vi "Module - Developer.vi"(11 "Stop":bool) -> (0 "Error Out":errorcluster)   [LabVIEW 2020]
uses:
  Control/Header - Select List Module.ctl
  Control/State - Module Developer.ctl
  <vilib>/Utility/miscctls.llb/LVPointTypeDef.ctl
  <vilib>/Utility/miscctls.llb/LVRowAndColumnUnsignedTypeDef.ctl
  <vilib>/Utility/miscctls.llb/LVPositionTypeDef.ctl
  <vilib>/Utility/miscctls.llb/LVRowAndColumnTypeDef.ctl
  Control/State - eFGV.ctl
  Control/Page List Configuration.ctl
  <vilib>/Utility/sysdir.llb/System Directory Type.ctl
  4b85dc79-c13a-48f8-9fb5-d693e32ae90e.vi
  de5a3265-ad59-4465-a9dd-367ad4980a1d.vi
  9e867a0b-6b5b-460c-ac8a-66f89ab5f6ca.vi
  ea73c07c-52c5-4c90-b3f8-ef615bf6d849.vi
  6d7569e3-b217-40ce-8343-143ededf8619.vi
  <vilib>/Utility/file.llb/Read Delimited Spreadsheet (string).vi
panel:
  in  "Page":enum32{"Page 1", "Page 2", "Page 3", "Page 4"}(radio)
  in  "Refresh":bool
  out "Max":i32
  in  "RT: Select All List":bool caption="Select All"
  in  "RT: Select All Module":bool caption="Select All"
  in  "Tab Control":enum32{"Page 1", "Page 2", "Page 3", "Page 4"}(tab)
  in  "HMI: Project Name":string caption="Project Name:"
  in  "HMI State":T1(ring)=enum."Maximized"
  in  "HMI: Check License":bool caption="Check License"
  in  "HMI: EXE Name":string caption="EXE Name:"
  in  "Page List":i32(listbox)
  in  "HMI: Version":enum16{"Demo", "User"}(ring) caption="Version"
  in  "HMI: Min Page":i32=2 caption="Minimum Page" min=2 max=8
  in  "HMI: Max Page":enum16{"4", "5", "6", "7", "8", "9"}(ring) caption="Maximum Page"
  out "No":i32[](array[numeric])=[1, 2, 3, 4, 5, 6, 7, 8, 9, 10, 11, 12, 13, 14, 15, 16, 17, 18, 19, 20, 21, 22, 23, 24, 25]
  in  "Res: Width":i16=1356
  in  "Res: Height":i16=655
  in  "Font Size":u32=44
  in  "License Level":T2(ring)=enum."Level 2"
  in  "License Type":T3(ring)=enum."Perpetual"
  in  "HMI: Default":bool
  in  "HMI: Select List":T4=enum."2 Default Run Module" caption="Select List"
  in  "Tip Strip":string caption="Set Button Tip Strip"
  in  "HMI: List":cluster{"Module Name":string, "Selected":bool}[](array[cluster])
  in  "Text":string caption="Set Button Text"
  in  "HMI: Update Text":bool
  in  "Table: Button Text":i32(listbox)
  in  "HMI: Down":bool
  in  "HMI: Up":bool
  in  "HMI: Sort":bool
  in  "HMI: Add":bool
  in  "HMI: Remove":bool
  in  "HMI: All Module":cluster{"Module Name":string, "Selected":bool}[](array[cluster]) caption="All Module"
  in  "HMI: Select All Module":bool caption="Select All"
  in  "RT: All Module":cluster{"Module Name":string, "Selected":bool}[](array[cluster])
  in  "RT: List":cluster{"Module Name":string, "Selected":bool}[](array[cluster])
  in  "RT: Add":bool
  in  "RT: Remove":bool
  in  "RT: Up":bool
  in  "RT: Down":bool
  in  "Load Error":bool
  in  "Error Table":i32(listbox) caption="List of Error"
  # "Page List"
  # "General Setting"
  # "Configure List of HMI Module"
  # "Configure Button Text"
  # "Maximum 15 page configurable"
  # "Configure List of RT Engine Module"
  # "Error Management"
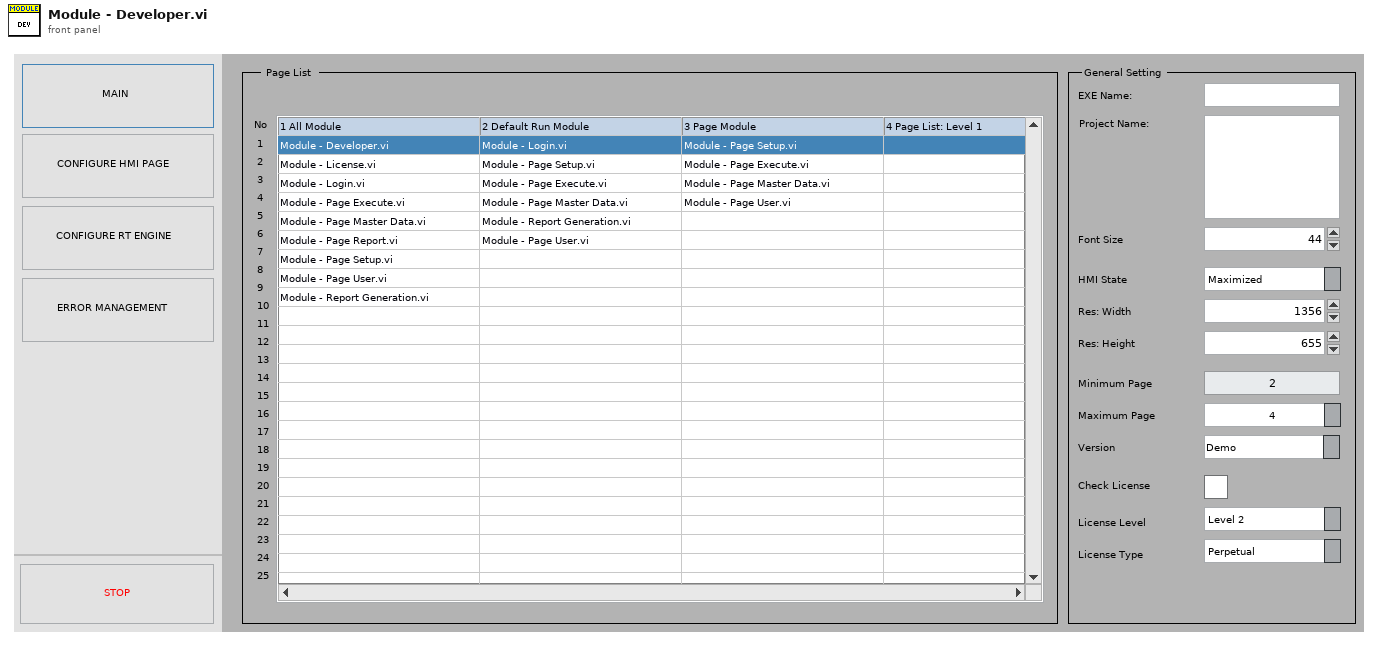
[diagram p1: front panel]
types:
  T1 = enum32{"Invalid", "Standard", "Closed", "Hidden", "Minimized", "Maximized"}
  T2 = enum32{"Level 1", "Level 2", "Level 3", "Level 4", "Level 5"}
  T3 = enum32{"Free", "Trial", "Subscription", "Perpetual"}
  T4 = typedef "Header - Select List Module.ctl" = enum16{"1 All Module", "2 Default Run Module", "3 Page Module", "4 Page List: Level 1", "5 Page List: Level 2", "6 Page List: Level 3", "7 All RT Module", "8 Default RT Run Module", "9 Acquire Enable Page", "10 Log Enable Page", "11 Run Page", "12 Kill Page", "13 Button Text", "14 Button Tip Strip"}
  T5 = cluster{"HMI?":bool, "HMI":cluster{"Button Ref":refnum<vi>[], "All Module":string[], "Button Disabled":enum8{"Enabled", "Disabled", "Disabled and Grayed Out"}[], "List From":enum16{"All HMI", "List HMI"}, "List Select":bool[]}, "RT":cluster{"Button Ref":refnum<vi>[], "All Module":string[], "Button Disabled":enum8{"Enabled", "Disabled", "Disabled and Grayed Out"}[], "List From":enum16{"All RT", "List RT"}, "List Select":bool[]}, "Event Ref":refnum<event-registration>}
  T6 = typedef "State - Module Developer.ctl" = enum16{"Init", "Register Event", "Get All Module", "Populate Page List", "Populate RT Module", "Idle", "HMI: List Disable", "HMI: Button Disable", "HMI: Update List", "HMI: Update Text Button", "HMI: Add to List", "HMI: Remove from List", "HMI: Sort List", "HMI: Up List", "HMI: Down List", "HMI: Set Default List", "RT: Add to List", "RT: Remove from List", "RT: Up List", "RT: Down List", "RT: List Disable", "RT: Button Disable", "Update Page List", "Save Page List", "Load Error", "Close"}
  T7 = typedef "LVPointTypeDef.ctl" = cluster{"Horizontal":i16, "Vertical":i16}
  T8 = typedef "LVPositionTypeDef.ctl" = cluster{"Left":i32, "Top":i32}
  T9 = typedef "LVRowAndColumnUnsignedTypeDef.ctl" = cluster{"Row":u32, "Column":u32}
  T10 = typedef "LVRowAndColumnTypeDef.ctl" = cluster{"Row":i32, "Column":i32}
  T11 = typedef "State - eFGV.ctl" = enum16{"Init", "Read", "Write", "Exit"}
  T12 = enum16{"Always On", "Always Off", "Off While Running"}
  T13 = enum8{"Enabled", "Disabled", "Disabled and Grayed Out"}
  T14 = typedef "Page List Configuration.ctl" = cluster{"HMI Configuration":cluster{"EXE Name":string, "Project Name":string, "Max Page No":i32, "HMI State":enum32{"Invalid", "Standard", "Closed", "Hidden", "Minimized", "Maximized"}, "Version":enum16{"Demo", "User"}, "Check License":bool, "Font Size":u32, "Res: Height":i16, "Res: Width":i16, "License Level":enum16{"Level 1", "Level 2", "Level 3", "Level 4", "Level 5"}, "License Type":enum16{"Free", "Trial", "Subscription", "Perpetual"}}, "All HMI Module":string[], "Default HMI Module":string[], "Page Module":string[], "Page List: Level 1":string[], "Page List: Level 2":string[], "Page List: Level 3":string[], "All RT Module":string[], "Default RT Module":string[], "Acquire Enable Page":string[], "Log Enable Page":string[], "Run Page":string[], "Kill Page":string[], "Button":cluster{"Text":string[], "Tip Strip":string[]}}
  T15 = enum32{"invalid app kind", "Development System", "Run Time System", "Student Edition", "Embedded LabVIEW", "Evaluation", "Custom"}
  T16 = enum16{"Free", "Trial", "Subscription", "Perpetual"}
  T17 = enum16{"Level 1", "Level 2", "Level 3", "Level 4", "Level 5"}
  T18 = enum8{"Enabled", "Disabled", "Disabled and Grayed Out"}[]
  T19 = typedef "System Directory Type.ctl" = i32
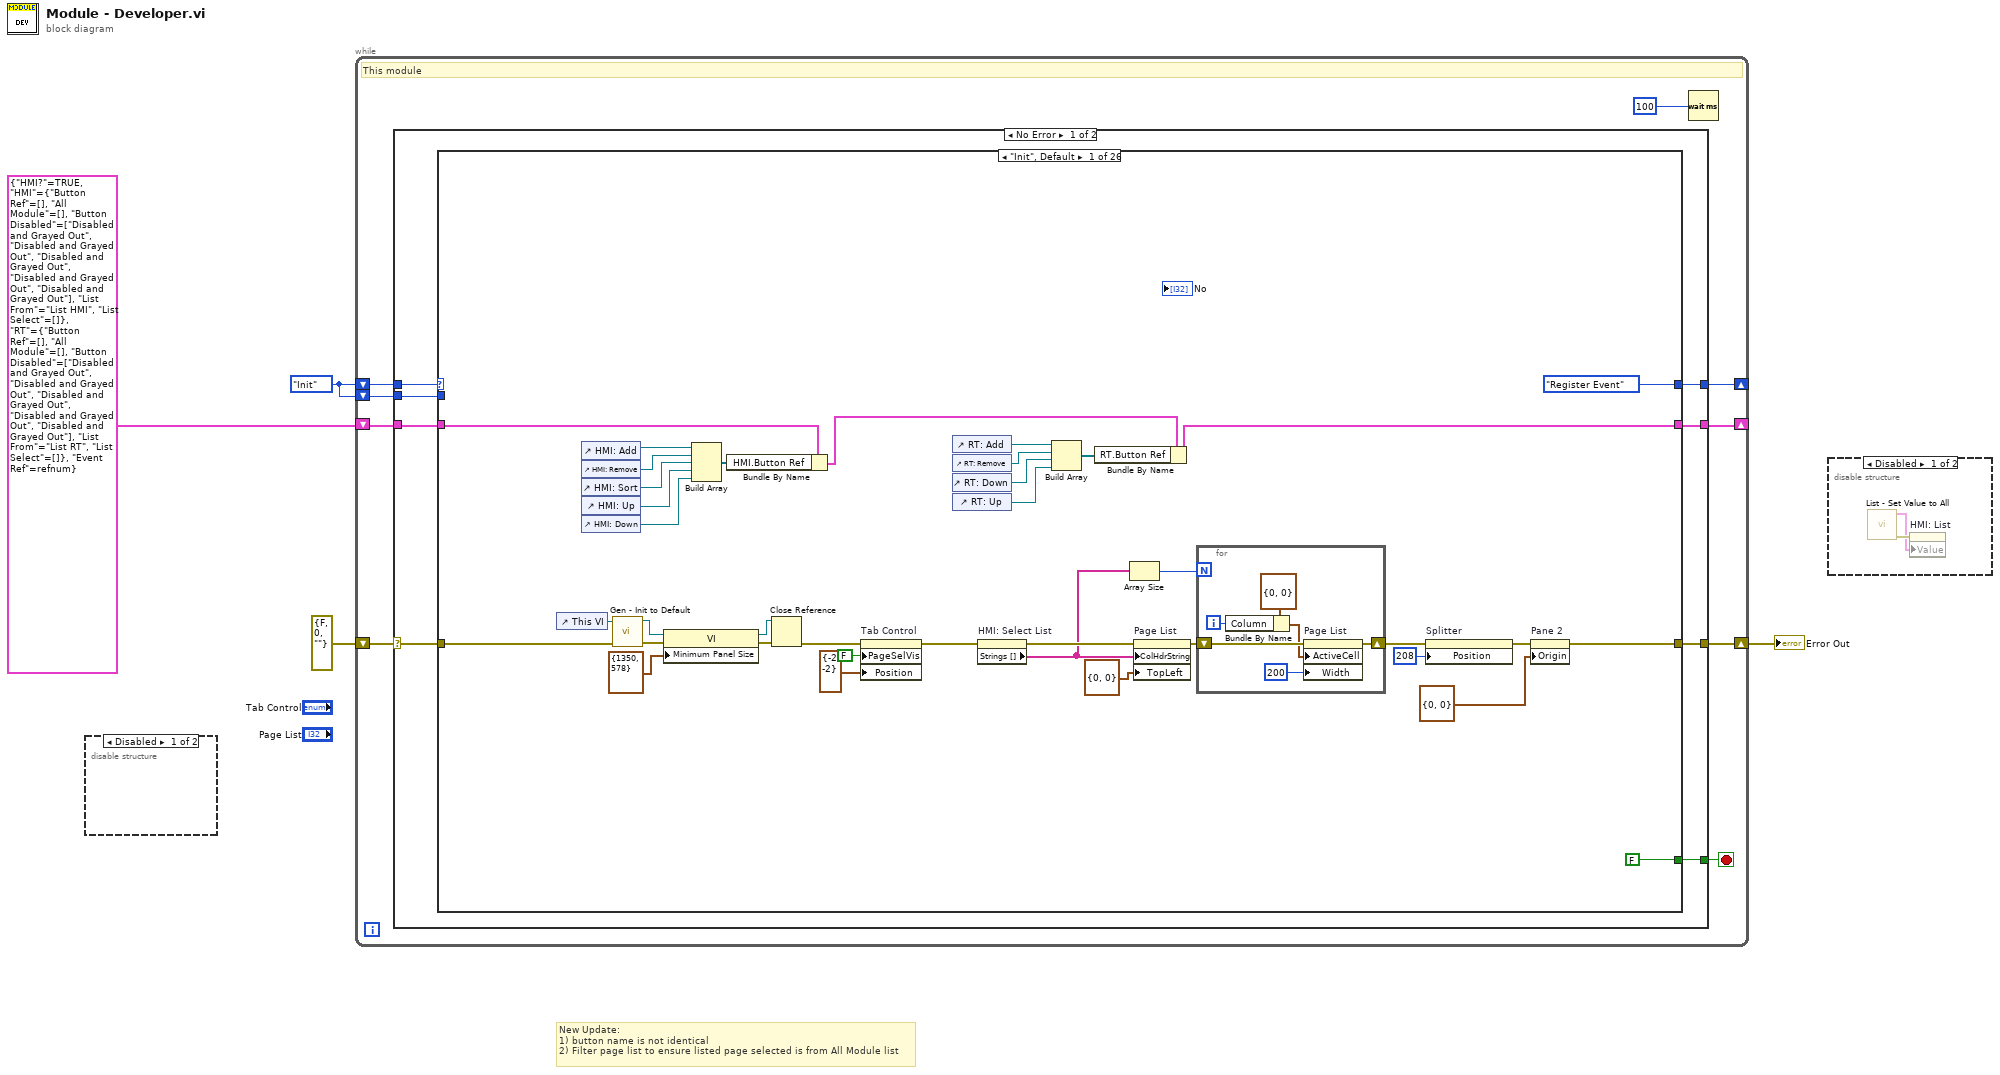
[diagram p0: block diagram]
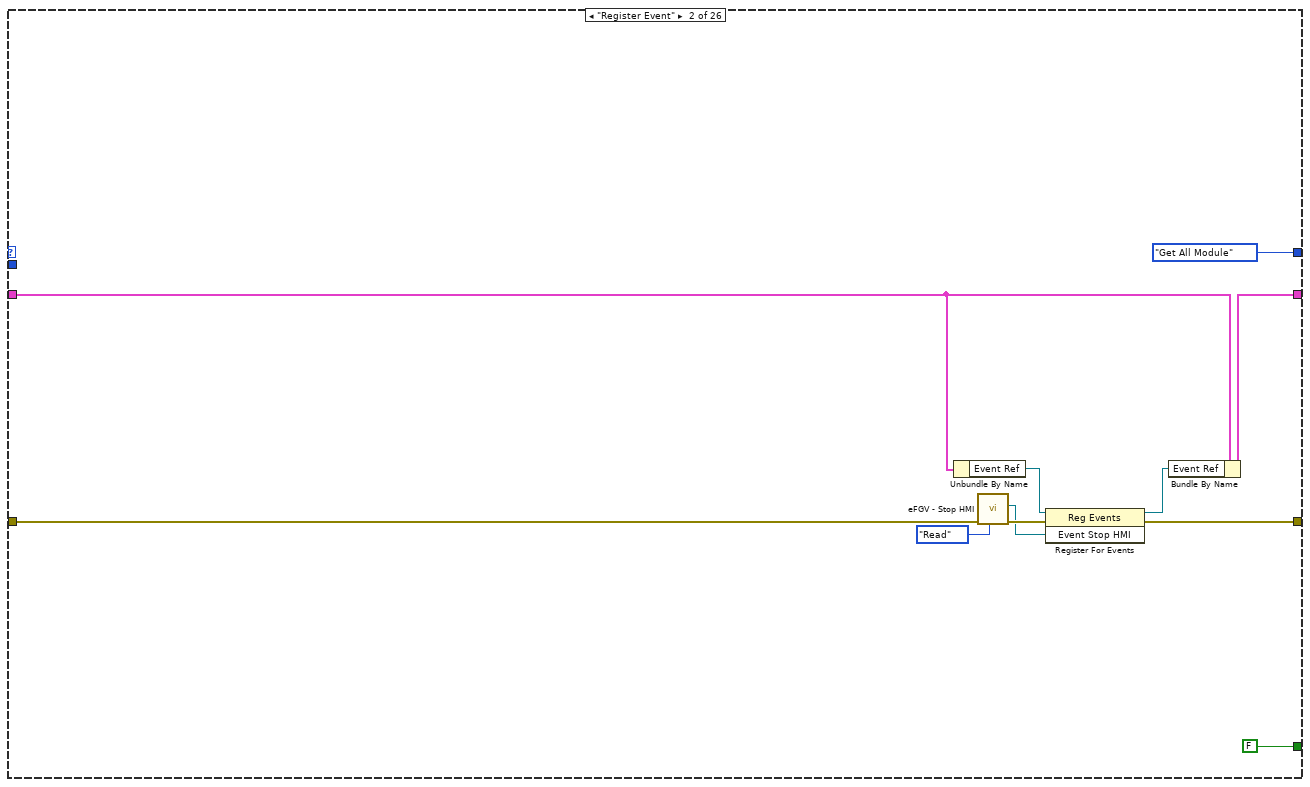
[diagram p4: hidden frame]
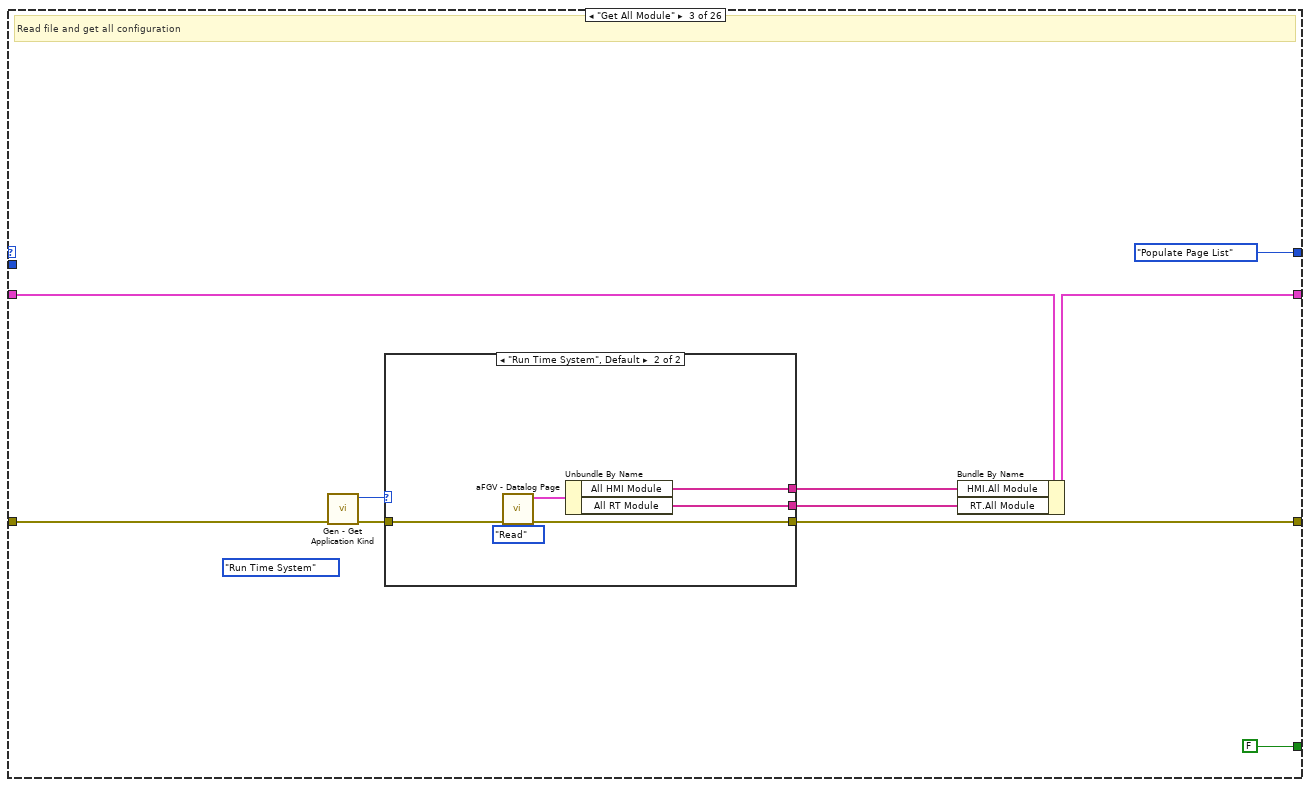
[diagram p5: hidden frame]
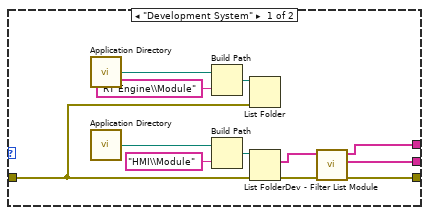
[diagram p6: hidden frame]
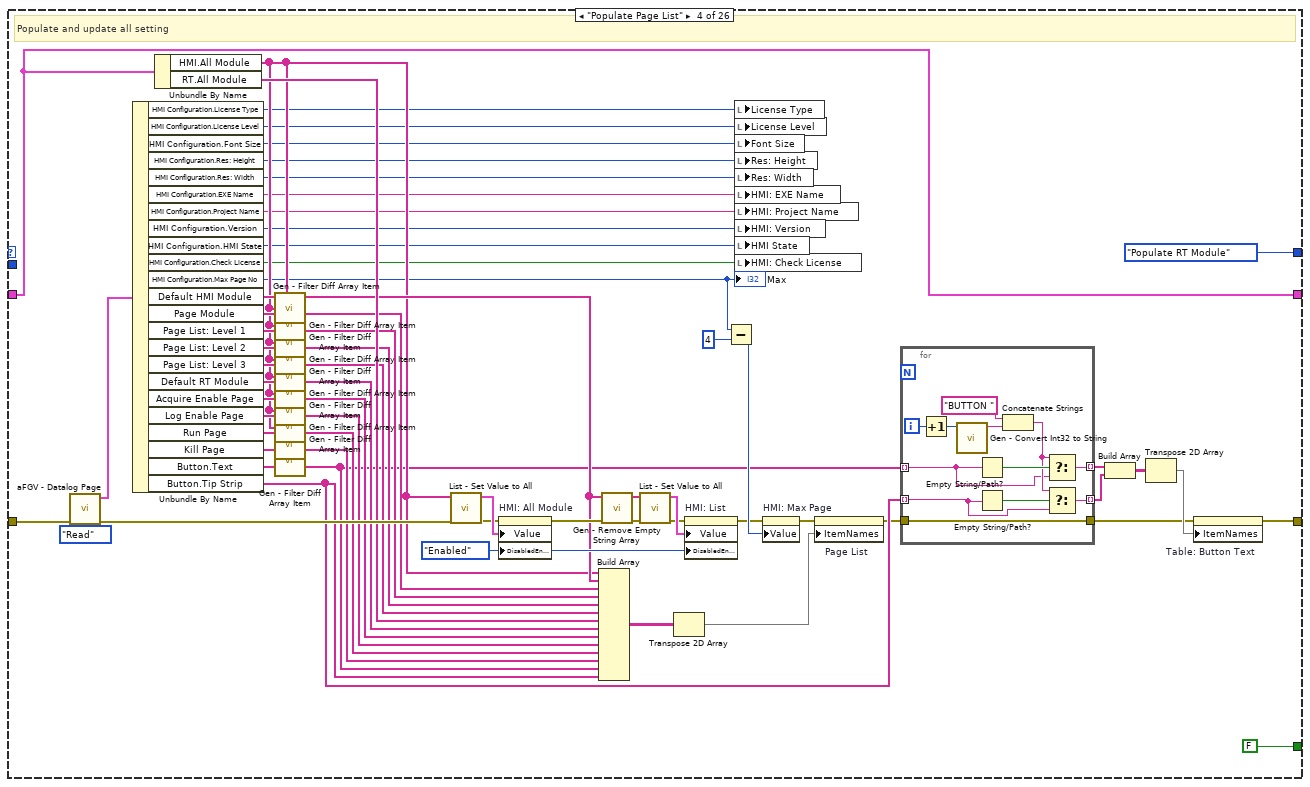
[diagram p7: hidden frame]
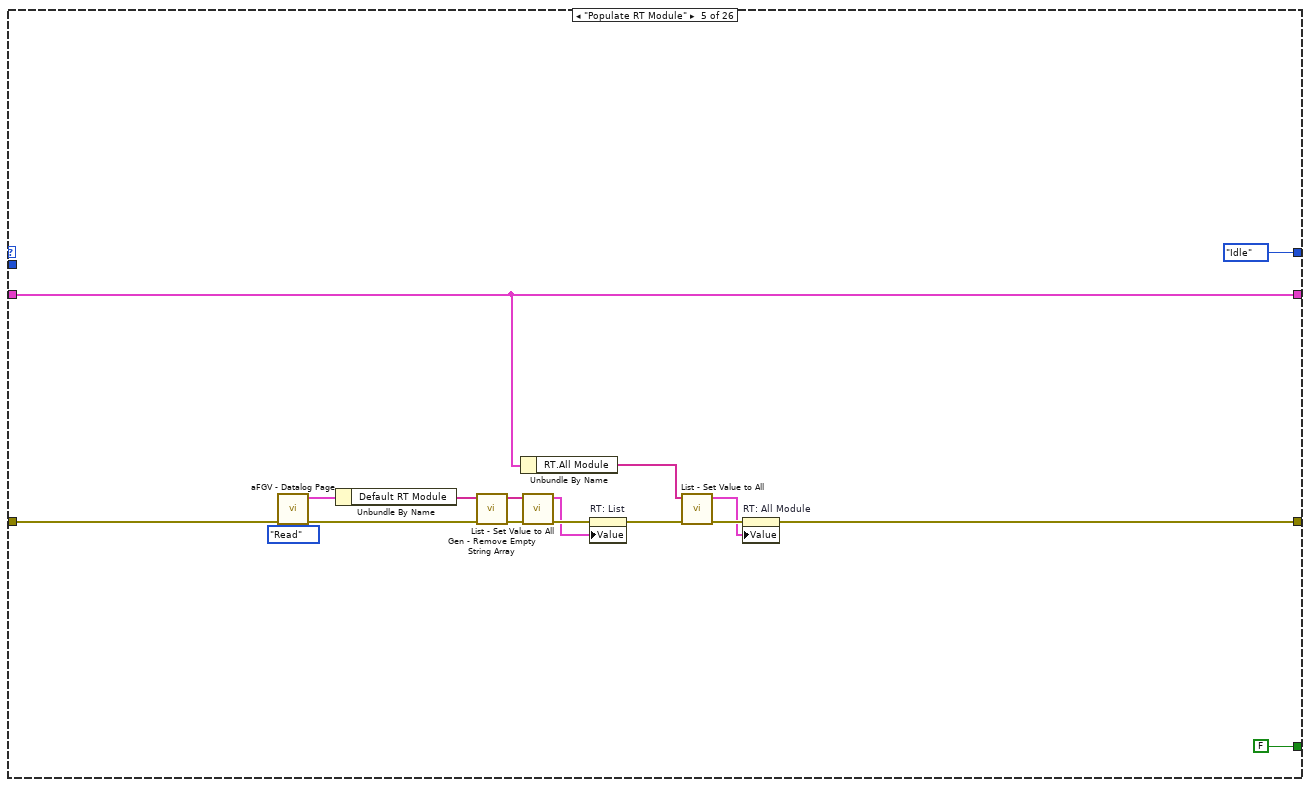
[diagram p8: hidden frame]
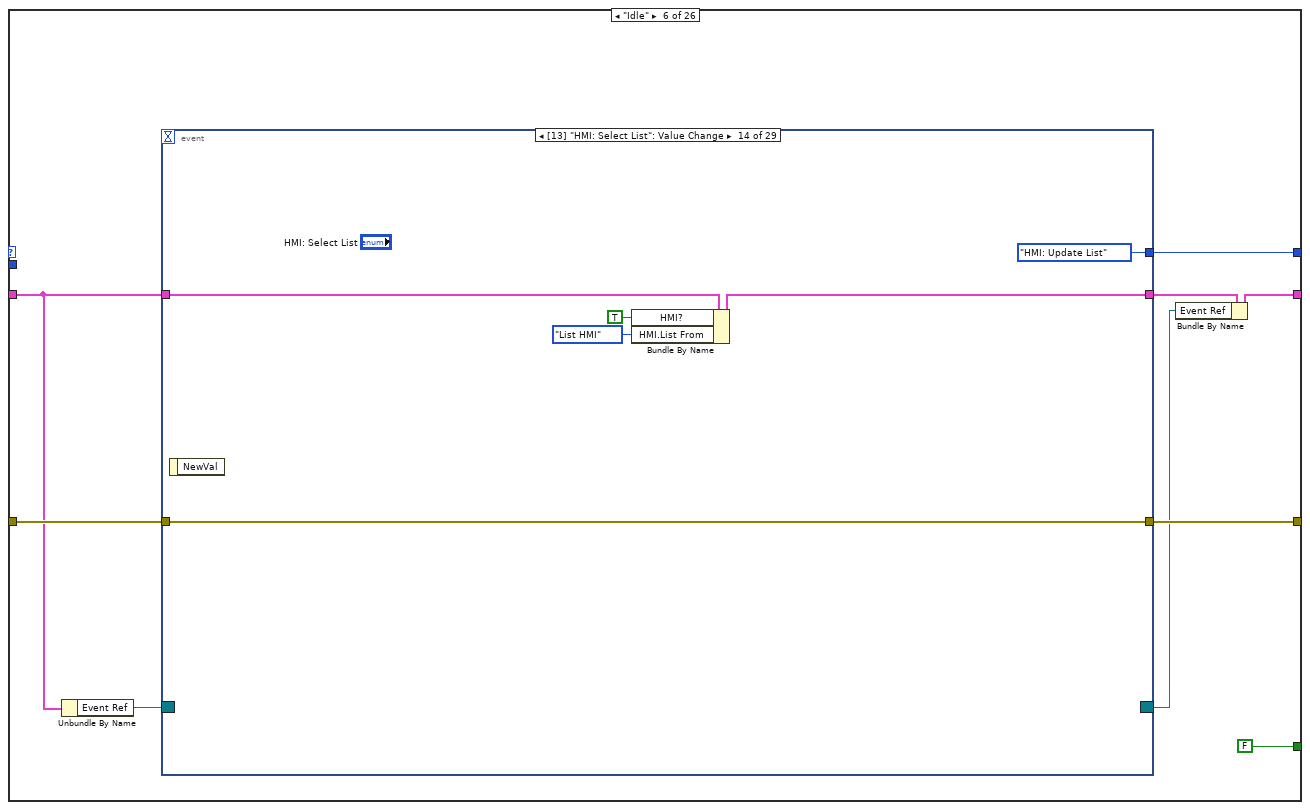
[diagram p9: hidden frame]
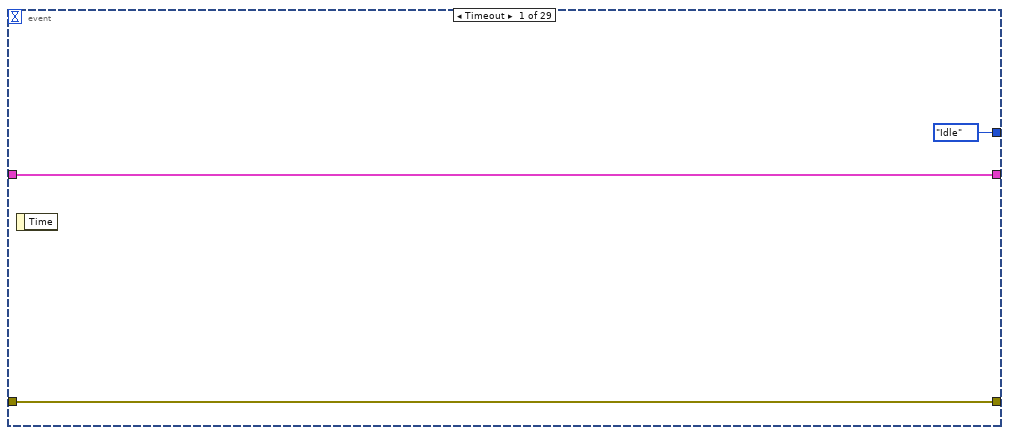
[diagram p10: hidden frame]
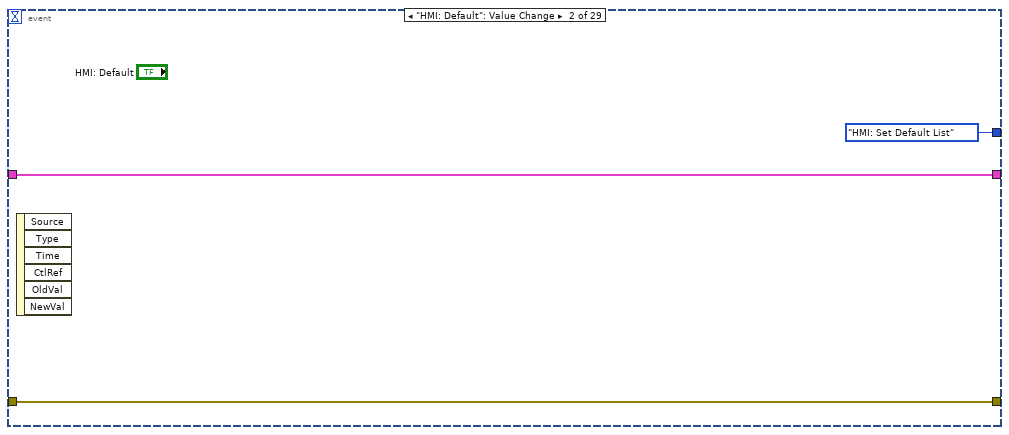
[diagram p11: hidden frame]
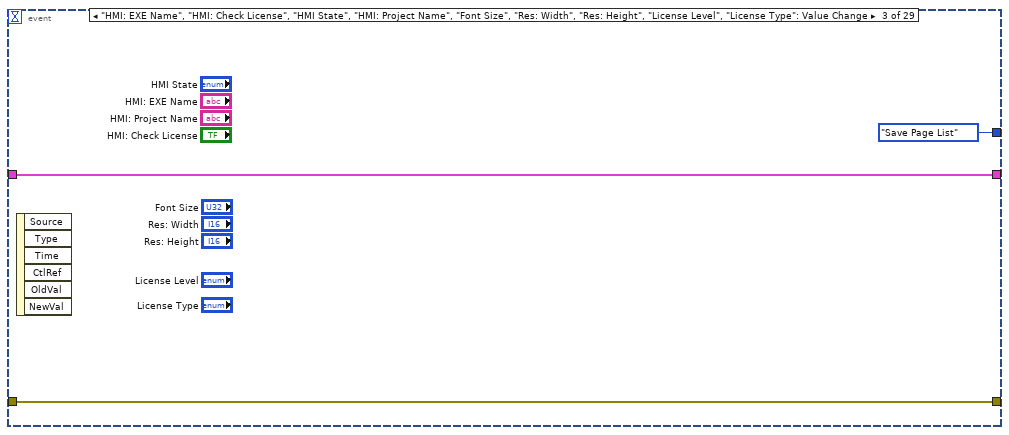
[diagram p12: hidden frame]
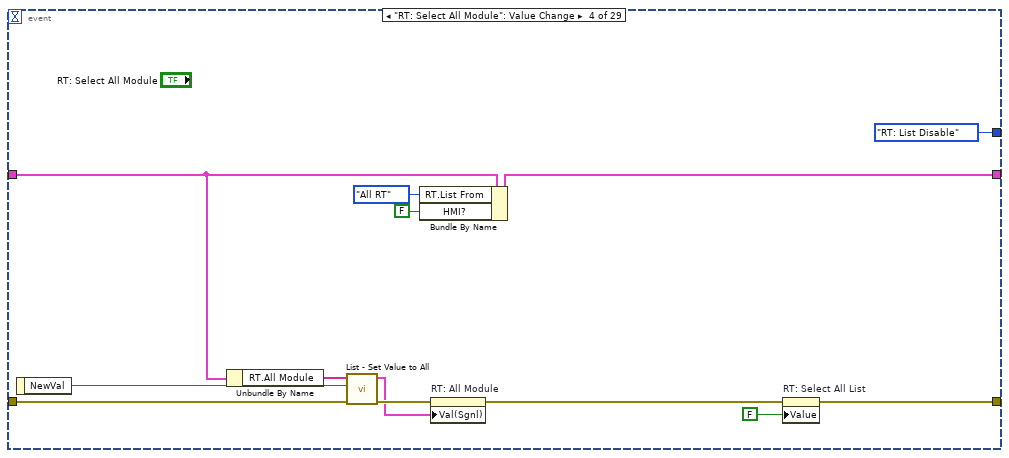
[diagram p13: hidden frame]
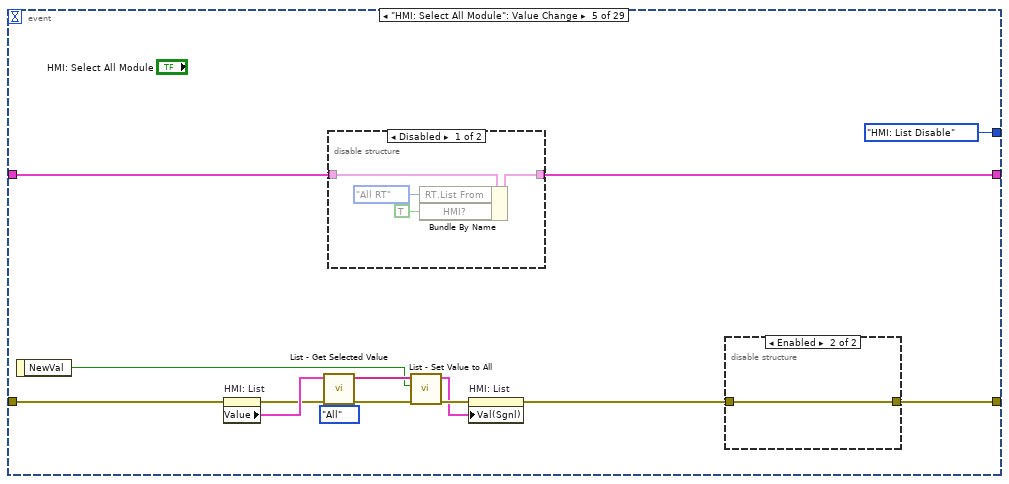
[diagram p14: hidden frame]
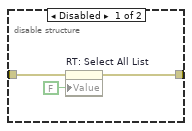
[diagram p15: hidden frame]
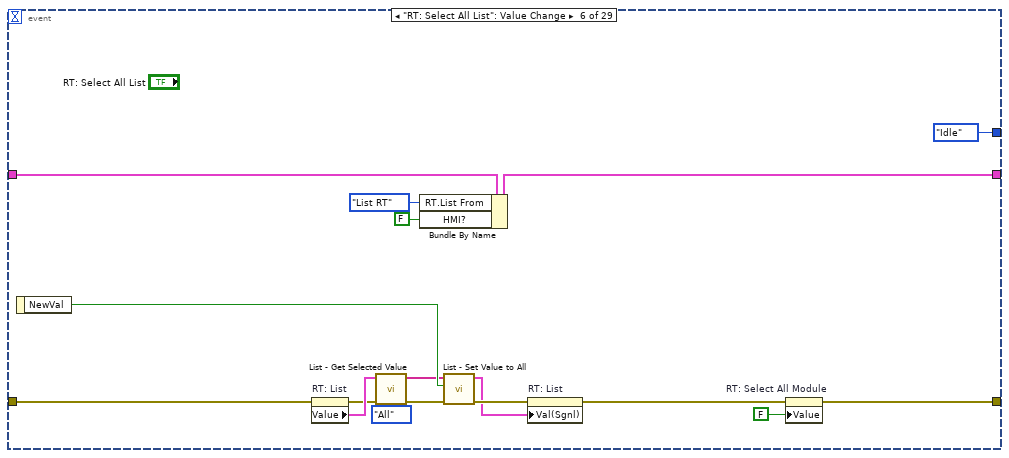
[diagram p17: hidden frame]
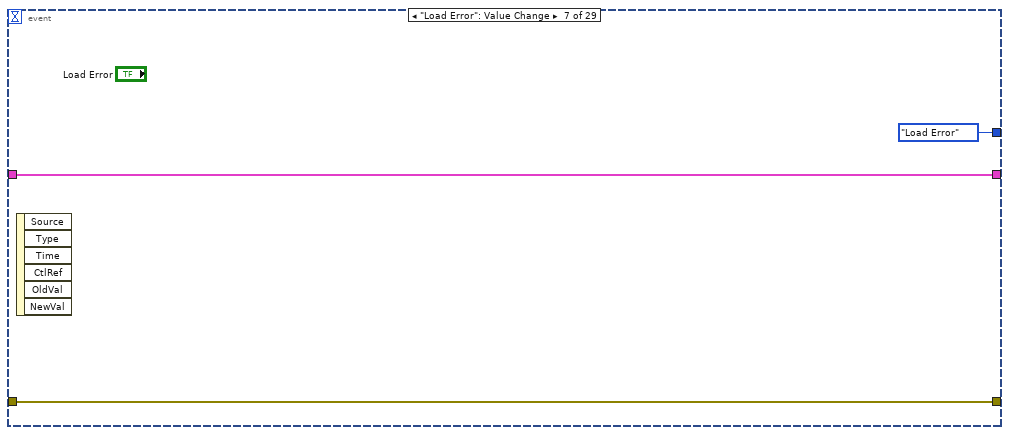
[diagram p18: hidden frame]
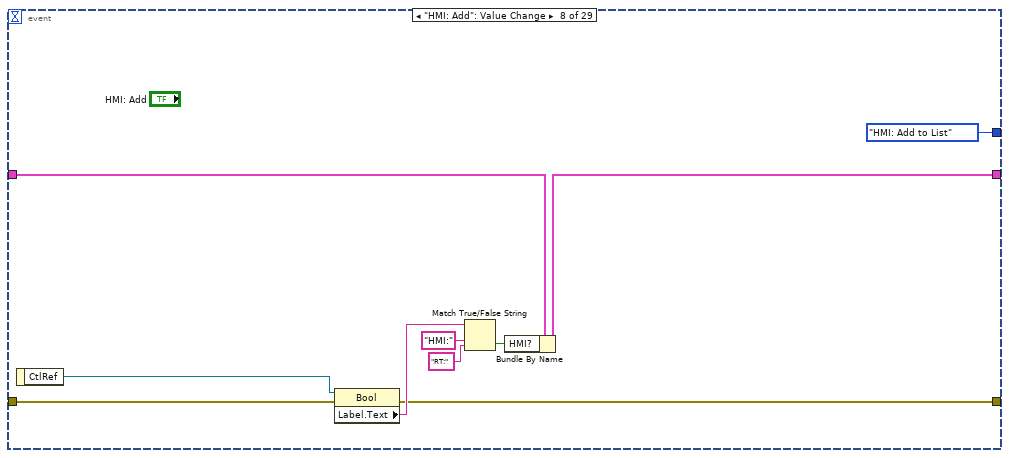
[diagram p19: hidden frame]
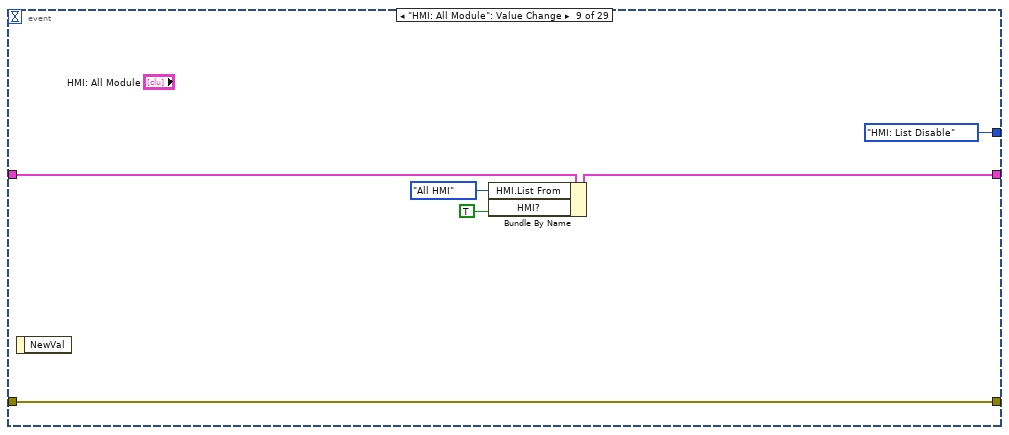
[diagram p20: hidden frame]
diagram:
  w1 = State_-_Module_Developer."Init"
  # "New Update:\n1) button name is not identical\n2) Filter page list to ensure listed page selected is from All Module list"
  n1 = disable-structure shown="Disabled" {
    frame Disabled {
    }
    frame Enabled {
    }
  }
  n2 = while {
    shift-right: [w9] -> _
    shift-left: w1 -> [w11]
    shift-right: [w12] -> w3
    shift-left: errorcluster {"status"=FALSE, "code"=0, "source"=""} ("Error In") -> [w13]
    shift-right: [w7] -> _
    shift-left: T5 {"HMI?"=TRUE, "HMI"={"Button Ref"=[], "All Module"=[], "Button Disabled"=[enum."Disabled and Grayed Out", enum."Disabled and Grayed Out", enum."Disabled and Grayed Out", enum."Disabled and Grayed Out", enum."Disabled and Grayed Out"], "List From"=enum."List HMI", "List Select"=[]}, "RT"={"Button Ref"=[], "All Module"=[], "Button Disabled"=[enum."Disabled and Grayed Out", enum."Disabled and Grayed Out", enum."Disabled and Grayed Out", enum."Disabled and Grayed Out", enum."Disabled and Grayed Out"], "List From"=enum."List RT", "List Select"=[]}, "Event Ref"=refnum} -> [w8]
    shift-left: w1 -> [w5]
    stop <- w10 stop-if-true
    # "This module"
    n3 = case shown="No Error" w13 {
      selector: w13 -> [w20 w1068]
      tunnel: w11 -> [w19 w1070]
      tunnel: [w21 w1067] -> w12
      tunnel: [w18 FALSE] -> w10
      tunnel: [w17 w1070] -> w9
      tunnel: w8 -> [w16 w1069]
      tunnel: [w15 w1069] -> w7
      tunnel: w5 -> [w14 _]
      frame No Error {
        n4 = case shown="\"Init\", Default" w19 {
          tunnel: [w32 w75 w82 w149 w178 w202 w440 w496 w530 w565 w639 w649 w674 w685 w710 w725 w766 w775 w784 w809 w822 w900 w923 w1015 w1019 w1056] -> w21
          tunnel: w20 -> [w58 w73 w79 w156 w190 w201 w439 w489 w529 w580 w633 w657 w675 w695 w714 w724 w758 w776 w794 w813 w834 w878 w908 w957 w1020 w1061]
          tunnel: [FALSE FALSE FALSE FALSE FALSE FALSE FALSE FALSE FALSE FALSE FALSE FALSE FALSE FALSE FALSE FALSE FALSE FALSE FALSE FALSE FALSE FALSE FALSE FALSE FALSE TRUE] -> w18
          tunnel: [State_-_Module_Developer."Register Event" State_-_Module_Developer."Get All Module" State_-_Module_Developer."Populate Page List" State_-_Module_Developer."Populate RT Module" State_-_Module_Developer."Idle" w199 State_-_Module_Developer."HMI: Button Disable" State_-_Module_Developer."Idle" State_-_Module_Developer."HMI: List Disable" State_-_Module_Developer."Save Page List" State_-_Module_Developer."Update Page List" State_-_Module_Developer."Update Page List" State_-_Module_Developer."Save Page List" State_-_Module_Developer."Update Page List" State_-_Module_Developer."Update Page List" State_-_Module_Developer."Update Page List" State_-_Module_Developer."Update Page List" State_-_Module_Developer."Update Page List" State_-_Module_Developer."Update Page List" State_-_Module_Developer."Update Page List" State_-_Module_Developer."RT: Button Disable" State_-_Module_Developer."Idle" State_-_Module_Developer."Save Page List" w953 State_-_Module_Developer."Idle" State_-_Module_Developer."Close"] -> w17
          tunnel: w16 -> [w57 w68 w85 w148 w189 w197 w454 w495 w539 w588 w640 w664 w681 w700 w722 w743 w769 w783 w799 w821 w847 w899 w928 w1017 w1033 w1055]
          tunnel: [w27 w66 w81 w148 w189 w195 w436 w495 w539 w588 w640 w664 w681 w700 w722 w743 w769 w783 w799 w821 w831 w899 w928 w1017 w1033 w1055] -> w15
          tunnel: w14 -> [_ _ _ _ _ _ _ _ _ _ _ _ _ _ _ _ _ _ _ _ _ _ _ _ _ _]
          frame "Init", Default {
            n5 = control-ref of="This VI"() -> (w51:refnum<vi>)
            n6 = control-ref of="HMI: Add"() -> (w50:refnum<vi>)
            n7 = control-ref of="HMI: Remove"() -> (w49:refnum<vi>)
            n8 = control-ref of="HMI: Sort"() -> (w48:refnum<vi>)
            n9 = control-ref of="HMI: Up"() -> (w47:refnum<vi>)
            n10 = control-ref of="HMI: Down"() -> (w46:refnum<vi>)
            n11 = call "Gen - Init to Default.vi"("Error in"=w58, "This VI"=w51) -> ("Error out"=w33:errorcluster, "This VI Copy"=w34:refnum<vi>)  [unwired: 8 in]
            n12 = property class="VI"(reference=w34, error in=w33, "Minimum Panel Size"=T7 {"Horizontal"=1350, "Vertical"=578} ("Front Panel Window:Minimum Size")) -> (reference out=w36:refnum<vi>, error out=w37:errorcluster)
            n13 = Build Array(w50, w49, w48, w47, w46) -> (w44:refnum<vi>[])
            n14 = Bundle By Name(cluster=w57, "HMI.Button Ref"=w44) -> (w45:T5)
            n15 = Close Reference(reference=w36, error in (no error)=w37) -> (error out=w23:errorcluster)
            n16 = property on="Tab Control" class="TabCtl (strict)"(error in=w23, "PageSelVis"=FALSE ("Page Selector Visible"), "Position"=T8 {"Left"=-2, "Top"=-2}) -> (error out=w22:errorcluster)  [unwired: 1 in, 1 out]
            n17 = control-ref of="RT: Add"() -> (w31:refnum<vi>)
            n18 = control-ref of="RT: Remove"() -> (w30:refnum<vi>)
            n19 = control-ref of="RT: Down"() -> (w29:refnum<vi>)
            n20 = control-ref of="RT: Up"() -> (w28:refnum<vi>)
            n21 = property on="HMI: Select List" class="Enum (strict)"(error in=w22) -> (error out=w25:errorcluster, "Strings []"=w24:string[])  [unwired: 1 in, 1 out]
            n22 = Build Array(w31, w30, w29, w28) -> (w26:refnum<vi>[])
            n23 = Bundle By Name(cluster=w45, "RT.Button Ref"=w26) -> (w27:T5)
            n24 = Array Size(array=w24) -> (size(s)=w42:i32)
            n25 = property on="Page List" class="MCListbox (strict)"(error in=w25, "ColHdrString"=w24, "TopLeft"=T9 {"Row"=0, "Column"=0} ("Top Left Visible Cell")) -> (error out=w43:errorcluster)  [unwired: 1 in, 1 out]
            n26 = for {
              N: w42 -> [_]
              shift-right: [w63] -> w41
              shift-left: w43 -> [w64]
              i -> [w60]
              n27 = Bundle By Name(cluster=T10 {"Row"=0, "Column"=0} ("Active Cell:Active Cell"), "Column"=w60) -> (w61:T10)
              n28 = property on="Page List" class="MCListbox (strict)"(error in=w64, "ActiveCell"=w61, "Width"=u32 200 ("Active Cell:Cell Size:Width")) -> (error out=w63:errorcluster)  [unwired: 1 in, 1 out]
            }
            n29 = property on="Splitter" class="Splitter"(error in=w41, "Position"=208 ("Splitter Position")) -> (error out=w53:errorcluster)  [unwired: 1 in, 1 out]
            n30 = property on="Pane 2" class="Pane"(error in=w53, "Origin"=T7 {"Horizontal"=0, "Vertical"=0}) -> (error out=w32:errorcluster)  [unwired: 1 in, 1 out]
          }
          frame "Register Event" {
            n31 = Unbundle By Name(w68) -> ("Event Ref"=w67:refnum<event-registration>)
            n32 = call "eFGV - Stop HMI.vi"("Action"=State_-_eFGV."Read", "Error In"=w73) -> ("Error Out"=w74:errorcluster, "Event Stop HMI"=w71:refnum<user-event>)  [unwired: 7 in, 1 out]
            n33 = register-events(reference=w67, error in=w74, w71) -> (reference out=w65:refnum<event-registration>, error out=w75:errorcluster)
            n34 = Bundle By Name(cluster=w68, "Event Ref"=w65) -> (w66:T5)
          }
          frame "Get All Module" {
            (unwired) T15."Run Time System" ("Application:Kind")
            # "Read file and get all configuration"
            n35 = call "Gen - Get Application Kind.vi"("Error In"=w79) -> ("Error Out"=w77:errorcluster, "Application:Kind"=w78:T15)  [unwired: 9 in]
            n36 = case shown="\"Run Time System\", Default" w78 {
              tunnel: [w86 w102] -> w82
              tunnel: w77 -> [w92 w103]
              tunnel: [w87 w99] -> w80
              tunnel: [w88 w98] -> w76
              frame "Development System" {
                n37 = call <vilib>:"Application Directory.vi"() -> ("Application Directory"=w94:path)
                n38 = call <vilib>:"Application Directory.vi"() -> ("Application Directory"=w95:path)
                n39 = Build Path(base path=w94, name or relative path="RT Engine\\Module") -> (appended path=w93:path)
                n40 = Build Path(base path=w95, name or relative path="HMI\\Module") -> (appended path=w96:path)
                n41 = List Folder(path=w93, error in=w92) -> ()  [unwired: 2 in, 4 out]
                n42 = List Folder(path=w96, error in=w92) -> (filenames=w89:string[], error out=w90:errorcluster)  [unwired: 2 in, 2 out]
                n43 = call "Dev - Filter List Module.vi"("Error In"=w90, "Module In"=w89) -> ("Error Out"=w86:errorcluster, "RT Module"=w87:string[], "HMI Module"=w88:string[])  [unwired: 7 in]
              }
              frame "Run Time System", Default {
                n44 = call "aFGV - Datalog Page.vi"("Action"=enum16{"Read", "Write"}."Read", "Error In"=w103) -> ("Error Out"=w102:errorcluster, "Data Out"=w100:T14)  [unwired: 8 in]
                n45 = Unbundle By Name(w100) -> ("All HMI Module"=w98:string[], "All RT Module"=w99:string[])
              }
            }
            n46 = Bundle By Name(cluster=w85, "HMI.All Module"=w76, "RT.All Module"=w80) -> (w81:T5)
          }
          frame "Populate Page List" {
            w136 = T13."Enabled" ("Disabled")
            # "Populate and update all setting"
            n47 = call "aFGV - Datalog Page.vi"("Action"=enum16{"Read", "Write"}."Read", "Error In"=w156) -> ("Error Out"=w165:errorcluster, "Data Out"=w157:T14)  [unwired: 8 in]
            n48 = Unbundle By Name(w157) -> ("HMI Configuration.License Type"=w104:T16, "HMI Configuration.License Level"=w105:T17, "HMI Configuration.Font Size"=w108:u32, "HMI Configuration.Res: Height"=w107:i16, "HMI Configuration.Res: Width"=w106:i16, "HMI Configuration.EXE Name"=w114:string, "HMI Configuration.Project Name"=w113:string, "HMI Configuration.Version"=w112:enum16{"Demo", "User"}, "HMI Configuration.HMI State"=w111:T1, "HMI Configuration.Check License"=w109:bool, "HMI Configuration.Max Page No"=w110:i32, "Default HMI Module"=w134:string[], "Page Module"=w164:string[], "Page List: Level 1"=w163:string[], "Page List: Level 2"=w162:string[], "Page List: Level 3"=w161:string[], "Default RT Module"=w146:string[], "Acquire Enable Page"=w147:string[], "Log Enable Page"=w154:string[], "Run Page"=w153:string[], "Kill Page"=w152:string[], "Button.Text"=w122:string[], "Button.Tip Strip"=w121:string[])
            "Max" <- w110
            n49 = Unbundle By Name(w148) -> ("HMI.All Module"=w123:string[], "RT.All Module"=w135:string[])
            n50 = call "Gen - Filter Diff Array Item.vi"("All Element"=w123, "List in"=w134) -> ("List Out"=w133:string[])  [unwired: 9 in]
            n51 = call "Gen - Filter Diff Array Item.vi"("All Element"=w123, "List in"=w164) -> ("List Out"=w132:string[])  [unwired: 9 in]
            n52 = call "Gen - Filter Diff Array Item.vi"("All Element"=w123, "List in"=w163) -> ("List Out"=w131:string[])  [unwired: 9 in]
            n53 = call "Gen - Filter Diff Array Item.vi"("All Element"=w123, "List in"=w162) -> ("List Out"=w130:string[])  [unwired: 9 in]
            n54 = call "Gen - Filter Diff Array Item.vi"("All Element"=w123, "List in"=w161) -> ("List Out"=w129:string[])  [unwired: 9 in]
            n55 = call "Gen - Filter Diff Array Item.vi"("All Element"=w123, "List in"=w146) -> ("List Out"=w128:string[])  [unwired: 9 in]
            n56 = call "Gen - Filter Diff Array Item.vi"("All Element"=w123, "List in"=w147) -> ("List Out"=w127:string[])  [unwired: 9 in]
            n57 = call "Gen - Filter Diff Array Item.vi"("All Element"=w123, "List in"=w154) -> ("List Out"=w126:string[])  [unwired: 9 in]
            n58 = call "Gen - Filter Diff Array Item.vi"("All Element"=w123, "List in"=w153) -> ("List Out"=w125:string[])  [unwired: 9 in]
            n59 = call "Gen - Filter Diff Array Item.vi"("All Element"=w123, "List in"=w152) -> ("List Out"=w124:string[])  [unwired: 9 in]
            n60 = call "List - Set Value to All.vi"("Error In"=w165, "List In"=w123) -> ("Error Out"=w142:errorcluster, "List Out"=w143:cluster{"Name":string, "Selected":bool}[])  [unwired: 8 in]
            n61 = property on="HMI: All Module" class="Arr (strict)"(error in=w142, "Value"=w143, "DisabledEnum"=w136) -> (error out=w138:errorcluster)  [unwired: 1 in, 1 out]
            n62 = Build Array(w123, w133, w132, w131, w130, w129, w135, w128, w127, w126, w125, w124, w122, w121) -> (w155:string[][])
            n63 = call "Gen - Remove Empty String Array.vi"("Data Array"=w133) -> ("Data Out"=w141:string[])  [unwired: 10 in]
            n64 = call "List - Set Value to All.vi"("Error In"=w138, "List In"=w141) -> ("Error Out"=w139:errorcluster, "List Out"=w140:cluster{"Name":string, "Selected":bool}[])  [unwired: 8 in]
            n65 = Transpose 2D Array(2D array=w155) -> (transposed array=w151:string[][])
            n66 = property on="HMI: List" class="Arr (strict)"(error in=w139, "Value"=w140, "DisabledEnum"=w136) -> (error out=w137:errorcluster)  [unwired: 1 in, 1 out]
            n67 = Subtract(x=w110, y=4) -> (x-y=w145:i32)
            n68 = local write "License Type"(w104) -> ()
            n69 = local write "License Level"(w105) -> ()
            n70 = local write "Font Size"(w108) -> ()
            n71 = local write "Res: Height"(w107) -> ()
            n72 = local write "Res: Width"(w106) -> ()
            n73 = local write "HMI: EXE Name"(w114) -> ()
            n74 = local write "HMI: Project Name"(w113) -> ()
            n75 = local write "HMI: Version"(w112) -> ()
            n76 = local write "HMI State"(w111) -> ()
            n77 = local write "HMI: Check License"(w109) -> ()
            n78 = property on="HMI: Max Page" class="Enum (strict)"(error in=w137, "Value"=w145) -> (error out=w150:errorcluster)  [unwired: 1 in, 1 out]
            n79 = property on="Page List" class="MCListbox (strict)"(error in=w150, "ItemNames"=w151) -> (error out=w115:errorcluster)  [unwired: 1 in, 1 out]
            n80 = for {
              tunnel: w122 -> [w169] mode=indexing
              tunnel: w121 -> [w166] mode=indexing
              tunnel: [w171] -> w120 mode=indexing
              tunnel: [w170] -> w119 mode=indexing
              tunnel: [w168] -> w116
              tunnel: w115 -> [w168]
              i -> [w167]
              n81 = Increment(x=w167) -> (x+1=w175:i32)
              n82 = call "Gen - Convert Int32 to String.vi"("Num In"=w175) -> ("String Out"=w173:string)  [unwired: 10 in]
              n83 = Empty String/Path?(string/path=w169) -> (empty?=w177:bool)
              n84 = Empty String/Path?(string/path=w166) -> (empty?=w176:bool)
              n85 = Concatenate Strings("BUTTON ", w173) -> (w172:string)
              n86 = Select(t=w172, s=w177, f=w169) -> (s? t:f=w171:string)
              n87 = Select(t=w172, s=w176, f=w166) -> (s? t:f=w170:string)
            }
            n88 = Build Array(w120, w119) -> (w118:string[][])
            n89 = Transpose 2D Array(2D array=w118) -> (transposed array=w117:string[][])
            n90 = property on="Table: Button Text" class="MCListbox (strict)"(error in=w116, "ItemNames"=w117) -> (error out=w149:errorcluster)  [unwired: 1 in, 1 out]
          }
          frame "Populate RT Module" {
            n91 = call "aFGV - Datalog Page.vi"("Action"=enum16{"Read", "Write"}."Read", "Error In"=w190) -> ("Error Out"=w179:errorcluster, "Data Out"=w184:T14)  [unwired: 8 in]
            n92 = Unbundle By Name(w184) -> ("Default RT Module"=w183:string[])
            n93 = call "Gen - Remove Empty String Array.vi"("Data Array"=w183) -> ("Data Out"=w188:string[])  [unwired: 10 in]
            n94 = Unbundle By Name(w189) -> ("RT.All Module"=w185:string[])
            n95 = call "List - Set Value to All.vi"("Error In"=w179, "List In"=w188) -> ("Error Out"=w186:errorcluster, "List Out"=w181:cluster{"Name":string, "Selected":bool}[])  [unwired: 8 in]
            n96 = property on="RT: List" class="Arr (strict)"(error in=w186, "Value"=w181) -> (error out=w182:errorcluster)  [unwired: 1 in, 1 out]
            n97 = call "List - Set Value to All.vi"("Error In"=w182, "List In"=w185) -> ("Error Out"=w187:errorcluster, "List Out"=w180:cluster{"Name":string, "Selected":bool}[])  [unwired: 8 in]
            n98 = property on="RT: All Module" class="Arr (strict)"(error in=w187, "Value"=w180) -> (error out=w178:errorcluster)  [unwired: 1 in, 1 out]
          }
          frame "Idle" {
            n99 = Unbundle By Name(w197) -> ("Event Ref"=w196:refnum<event-registration>)
            n100 = event shown="[13] \"HMI: Select List\": Value Change" {
              selector: w196 -> [_ _ _ _ _ _ _ _ _ _ _ _ _ _ _ _ _ _ _ _ _ _ _ _ _ _ _ _ _]
              dyn-events: [_ _ _ _ _ _ _ _ _ _ _ _ _ _ _ _ _ _ _ _ _ _ _ _ _ _ _ _ _] -> w194
              timeout: _ -> [_ _ _ _ _ _ _ _ _ _ _ _ _ _ _ _ _ _ _ _ _ _ _ _ _ _ _ _ _]
              tunnel: [w205 w208 w211 w217 w237 w253 w267 w269 w281 w292 w298 w303 w309 w317 w324 w333 w334 w343 w346 w359 w364 w370 w375 w381 w386 w391 w396 w424 w427] -> w202
              tunnel: w201 -> [w205 w208 w211 w221 w231 w261 w267 w268 w281 w292 w298 w304 w309 w317 w324 w333 w334 w343 w350 w359 w364 w370 w375 w381 w386 w391 w406 w424 w427]
              tunnel: [State_-_Module_Developer."Idle" State_-_Module_Developer."HMI: Set Default List" State_-_Module_Developer."Save Page List" State_-_Module_Developer."RT: List Disable" State_-_Module_Developer."HMI: List Disable" State_-_Module_Developer."Idle" State_-_Module_Developer."Load Error" State_-_Module_Developer."HMI: Add to List" State_-_Module_Developer."HMI: List Disable" w287 State_-_Module_Developer."HMI: List Disable" State_-_Module_Developer."Save Page List" State_-_Module_Developer."HMI: Remove from List" State_-_Module_Developer."HMI: Update List" State_-_Module_Developer."HMI: Sort List" w327 State_-_Module_Developer."HMI: Update Text Button" State_-_Module_Developer."Save Page List" State_-_Module_Developer."Idle" State_-_Module_Developer."Get All Module" State_-_Module_Developer."RT: Add to List" State_-_Module_Developer."RT: List Disable" State_-_Module_Developer."RT: Down List" State_-_Module_Developer."RT: List Disable" State_-_Module_Developer."RT: Remove from List" State_-_Module_Developer."RT: Up List" State_-_Module_Developer."Idle" State_-_Module_Developer."Close" State_-_Module_Developer."Close"] -> w199
              tunnel: [w204 w207 w210 w212 w235 w248 w266 w275 w280 w285 w295 w300 w311 w316 w321 w326 w336 w340 w352 w358 w361 w367 w372 w378 w383 w388 w408 w423 w426] -> w198
              tunnel: w197 -> [w204 w207 w210 w213 w236 w249 w266 w277 w283 w291 w297 w308 w313 w318 w323 w332 w338 w342 w352 w358 w363 w369 w374 w380 w385 w390 w408 w423 w426]
              event Timeout {
                n101 = event-data() -> ()  [unwired: 1 in, 1 out]
              }
              event "HMI: Default": Value Change {
                n102 = event-data() -> ()  [unwired: 1 in, 6 out]
              }
              event "HMI: EXE Name", "HMI: Check License", "HMI State", "HMI: Project Name", "Font Size", "Res: Width", "Res: Height", "License Level", "License Type": Value Change {
                n103 = event-data() -> ()  [unwired: 1 in, 6 out]
              }
              event "RT: Select All Module": Value Change {
                n104 = event-data() -> ("NewVal"=w222:bool)  [unwired: 1 in]
                n105 = Unbundle By Name(w213) -> ("RT.All Module"=w223:string[])
                n106 = call "List - Set Value to All.vi"("Error In"=w221, "Selected"=w222, "List In"=w223) -> ("Error Out"=w220:errorcluster, "List Out"=w219:cluster{"Name":string, "Selected":bool}[])  [unwired: 7 in]
                n107 = Bundle By Name(cluster=w213, "RT.List From"=enum16{"All RT", "List RT"}."All RT" ("RT: List From"), "HMI?"=FALSE) -> (w212:T5)
                n108 = property on="RT: All Module" class="Arr (strict)"(error in=w220, "Val(Sgnl)"=w219) -> (error out=w218:errorcluster)  [unwired: 1 in, 1 out]
                n109 = property on="RT: Select All List" class="Bool (strict)"(error in=w218, "Value"=FALSE ("RT: Select All List")) -> (error out=w217:errorcluster)  [unwired: 1 in, 1 out]
              }
              event "HMI: Select All Module": Value Change {
                n110 = event-data() -> ("NewVal"=w225:bool)  [unwired: 1 in]
                n111 = property on="HMI: List" class="Arr (strict)"(error in=w231) -> (error out=w230:errorcluster, "Value"=w233:cluster{"Module Name":string, "Selected":bool}[])  [unwired: 1 in, 1 out]
                n112 = call "List - Get Selected Value.vi"("Select"=enum16{"All", "True", "False"}."All", "Error In"=w230, "List In"=w233) -> ("Error Out"=w229:errorcluster, "List Out"=w226:string[])  [unwired: 7 in]
                n113 = disable-structure shown="Disabled" {
                  disable-tunnel: w236 -> [w244 w247]
                  disable-tunnel: [w243 w247] -> w235
                  frame Disabled {
                    n114 = Bundle By Name(cluster=w244, "RT.List From"=enum16{"All RT", "List RT"}."All RT" ("RT: List From"), "HMI?"=TRUE) -> (w243:T5)
                  }
                  frame Enabled {
                  }
                }
                n115 = call "List - Set Value to All.vi"("Error In"=w229, "Selected"=w225, "List In"=w226) -> ("Error Out"=w228:errorcluster, "List Out"=w227:cluster{"Name":string, "Selected":bool}[])  [unwired: 7 in]
                n116 = property on="HMI: List" class="Arr (strict)"(error in=w228, "Val(Sgnl)"=w227) -> (error out=w234:errorcluster)  [unwired: 1 in, 1 out]
                n117 = disable-structure shown="Enabled" {
                  disable-tunnel: [w241 w242] -> w237
                  disable-tunnel: w234 -> [w239 w242]
                  frame Disabled {
                    n118 = property on="RT: Select All List" class="Bool (strict)"(error in=w239, "Value"=FALSE ("RT: Select All List")) -> (error out=w241:errorcluster)  [unwired: 1 in, 1 out]
                  }
                  frame Enabled {
                  }
                }
              }
              event "RT: Select All List": Value Change {
                n119 = event-data() -> ("NewVal"=w259:bool)  [unwired: 1 in]
                n120 = property on="RT: List" class="Arr (strict)"(error in=w261) -> (error out=w258:errorcluster, "Value"=w260:cluster{"Module Name":string, "Selected":bool}[])  [unwired: 1 in, 1 out]
                n121 = call "List - Get Selected Value.vi"("Select"=enum16{"All", "True", "False"}."All", "Error In"=w258, "List In"=w260) -> ("Error Out"=w257:errorcluster, "List Out"=w256:string[])  [unwired: 7 in]
                n122 = Bundle By Name(cluster=w249, "RT.List From"=enum16{"All RT", "List RT"}."List RT" ("RT: List From"), "HMI?"=FALSE) -> (w248:T5)
                n123 = call "List - Set Value to All.vi"("Error In"=w257, "Selected"=w259, "List In"=w256) -> ("Error Out"=w263:errorcluster, "List Out"=w262:cluster{"Name":string, "Selected":bool}[])  [unwired: 7 in]
                n124 = property on="RT: List" class="Arr (strict)"(error in=w263, "Val(Sgnl)"=w262) -> (error out=w254:errorcluster)  [unwired: 1 in, 1 out]
                n125 = property on="RT: Select All Module" class="Bool (strict)"(error in=w254, "Value"=FALSE ("RT: Select All Module")) -> (error out=w253:errorcluster)  [unwired: 1 in, 1 out]
              }
              event "Load Error": Value Change {
                n126 = event-data() -> ()  [unwired: 1 in, 6 out]
              }
              event "HMI: Add": Value Change {
                n127 = event-data() -> ("CtlRef"=w274:refnum<vi>)  [unwired: 1 in]
                n128 = property class="Bool"(reference=w274, error in=w268) -> (error out=w269:errorcluster, "Label.Text"=w271:string)  [unwired: 1 out]
                n129 = Match True/False String(2:"RT:" ("false string"), 3:"HMI:" ("true string"), 4:w271) -> (0:w270:bool)  [unwired: 1 out]
                n130 = Bundle By Name(cluster=w277, "HMI?"=w270) -> (w275:T5)
              }
              event "HMI: All Module": Value Change {
                n131 = event-data() -> ()  [unwired: 1 in, 1 out]
                n132 = Bundle By Name(cluster=w283, "HMI.List From"=enum16{"All HMI", "List HMI"}."All HMI" ("List From"), "HMI?"=TRUE) -> (w280:T5)
              }
              event "HMI: Down": Value Change {
                n133 = event-data() -> ("Time"=w286:u32)  [unwired: 1 in]
                n134 = Bundle By Name(cluster=w291, "HMI?"=TRUE) -> (w285:T5)
                n135 = call "Gen - Check for Repeating User Event.vi"("Time"=w286) -> ("Repeat?"=w290:bool)  [unwired: 10 in]
                n136 = Select(t=State_-_Module_Developer."HMI: Down List", s=w290, f=State_-_Module_Developer."Idle") -> (s? t:f=w287:T6)
              }
              event "HMI: List": Value Change {
                n137 = event-data() -> ()  [unwired: 1 in, 6 out]
                n138 = Bundle By Name(cluster=w297, "HMI.List From"=enum16{"All HMI", "List HMI"}."List HMI" ("List From"), "HMI?"=TRUE) -> (w295:T5)
              }
              event "HMI: Max Page": Value Change {
                n139 = event-data() -> ()  [unwired: 1 in, 6 out]
                n140 = property on="HMI: Max Page" class="Enum (strict)"(error in=w304) -> (error out=w303:errorcluster, "Value"=w306:enum16{"4", "5", "6", "7", "8", "9"})  [unwired: 1 in, 1 out]
                n141 = To Long Integer(number=w306) -> (32bit integer=w305:i32)
                n142 = Add(x=w305, y=4) -> (x+y=w302:i32)
                n143 = local write "Max"(w302) -> ()
                n144 = Bundle By Name(cluster=w308, "HMI?"=TRUE) -> (w300:T5)
              }
              event "HMI: Remove": Value Change {
                n145 = event-data() -> ()  [unwired: 1 in, 6 out]
                n146 = Bundle By Name(cluster=w313, "HMI?"=TRUE) -> (w311:T5)
              }
              event Value Change {
                n147 = event-data() -> ()  [unwired: 1 in, 1 out]
                n148 = Bundle By Name(cluster=w318, "HMI?"=TRUE, "HMI.List From"=enum16{"All HMI", "List HMI"}."List HMI" ("List From")) -> (w316:T5)
              }
              event "HMI: Sort": Value Change {
                n149 = event-data() -> ()  [unwired: 1 in, 6 out]
                n150 = Bundle By Name(cluster=w323, "HMI?"=TRUE) -> (w321:T5)
              }
              event "HMI: Up": Value Change {
                n151 = event-data() -> ("Time"=w331:u32)  [unwired: 1 in]
                n152 = Bundle By Name(cluster=w332, "HMI?"=TRUE) -> (w326:T5)
                n153 = call "Gen - Check for Repeating User Event.vi"("Time"=w331) -> ("Repeat?"=w330:bool)  [unwired: 10 in]
                n154 = Select(t=State_-_Module_Developer."HMI: Up List", s=w330, f=State_-_Module_Developer."Idle") -> (s? t:f=w327:T6)
              }
              event "HMI: Update Text": Value Change {
                n155 = event-data() -> ()  [unwired: 1 in, 6 out]
                n156 = Bundle By Name(cluster=w338, "HMI?"=TRUE) -> (w336:T5)
              }
              event "HMI: Version": Value Change {
                n157 = event-data() -> ()  [unwired: 1 in, 1 out]
                n158 = Bundle By Name(cluster=w342, "HMI?"=TRUE) -> (w340:T5)
              }
              event "Page": Value Change {
                n159 = event-data() -> ("NewVal"=w349:enum32{"Page 1", "Page 2", "Page 3", "Page 4"})  [unwired: 1 in]
                n160 = property on="Tab Control" class="TabCtl (strict)"(error in=w350, "Value"=w349) -> (error out=w348:errorcluster)  [unwired: 1 in, 1 out]
                n161 = case shown="\"Page 1\", Default" w349 {
                  tunnel: [w354 w356] -> w347
                  tunnel: w348 -> [w354 w356]
                  tunnel: [T12."Always Off" ("Horizontal Scrollbar Visibility") T12."Always Off" ("Horizontal Scrollbar Visibility")] -> w345
                  frame "Page 1", Default {
                  }
                  frame "Page 2" {
                  }
                }
                n162 = property on="Pane 2" class="Pane"(error in=w347, "HorizScrollbarVisibility"=w345, "Origin"=T7 {"Horizontal"=0, "Vertical"=0}) -> (error out=w346:errorcluster)  [unwired: 1 in, 1 out]
              }
              event "Refresh": Value Change {
                n163 = event-data() -> ()  [unwired: 1 in, 6 out]
              }
              event "RT: Add": Value Change {
                n164 = event-data() -> ()  [unwired: 1 in, 6 out]
                n165 = Bundle By Name(cluster=w363, "HMI?"=FALSE) -> (w361:T5)
              }
              event "RT: All Module": Value Change {
                n166 = event-data() -> ()  [unwired: 1 in, 6 out]
                n167 = Bundle By Name(cluster=w369, "RT.List From"=enum16{"All RT", "List RT"}."All RT" ("RT: List From"), "HMI?"=FALSE) -> (w367:T5)
              }
              event "RT: Down": Value Change {
                n168 = event-data() -> ()  [unwired: 1 in, 6 out]
                n169 = Bundle By Name(cluster=w374, "HMI?"=FALSE) -> (w372:T5)
              }
              event "RT: List": Value Change {
                n170 = event-data() -> ()  [unwired: 1 in, 6 out]
                n171 = Bundle By Name(cluster=w380, "HMI?"=FALSE, "RT.List From"=enum16{"All RT", "List RT"}."List RT" ("RT: List From")) -> (w378:T5)
              }
              event "RT: Remove": Value Change {
                n172 = event-data() -> ()  [unwired: 1 in, 6 out]
                n173 = Bundle By Name(cluster=w385, "HMI?"=FALSE) -> (w383:T5)
              }
              event "RT: Up": Value Change {
                n174 = event-data() -> ()  [unwired: 1 in, 6 out]
                n175 = Bundle By Name(cluster=w390, "HMI?"=FALSE) -> (w388:T5)
              }
              event "Table: Button Text": Mouse Down {
                n176 = event-data() -> ()  [unwired: 1 in, 1 out]
                n177 = property on="Table: Button Text" class="MCListbox (strict)"(error in=w406) -> (error out=w400:errorcluster, "ItemNames"=w405:string[][], "SelectedCell"=w403:T10)  [unwired: 1 in, 1 out]
                n178 = Unbundle By Name(w403) -> ("Row"=w395:i32)
                n179 = In Range and Coerce(upper limit=15, x=w395, lower limit=0) -> (In Range?=w392:bool)  [unwired: 1 out]
                n180 = case shown="True" w392 {
                  tunnel: w405 -> [_ w421]
                  tunnel: [w413 w420] -> w404
                  tunnel: [w413 w417] -> w401
                  tunnel: w395 -> [_ w416]
                  tunnel: w400 -> [w410 w415]
                  tunnel: [w409 w415] -> w399
                  tunnel: [T13."Disabled and Grayed Out" ("Disabled") T13."Enabled" ("Disabled")] -> w397
                  frame False {
                    w413 = ""
                    n181 = property on="Table: Button Text" class="MCListbox (strict)"(error in=w410, "Value"=-1 ("Table: Button Text")) -> (error out=w409:errorcluster)  [unwired: 1 in, 1 out]
                  }
                  frame True {
                    n182 = Index Array(array=w421, index (row) #1=w416, index (col) #1=0 ("disabled index (col)"), index (row) #2=w416, index (col) #2=1 ("disabled index (col)")) -> (element #1=w420:string, element #2=w417:string)
                  }
                }
                n183 = property on="Text" class="Str"(error in=w399, "Value"=w404) -> (error out=w402:errorcluster)  [unwired: 1 in, 1 out]
                n184 = property on="Tip Strip" class="Str"(error in=w402, "Value"=w401) -> (error out=w398:errorcluster)  [unwired: 1 in, 1 out]
                n185 = property on="HMI: Update Text" class="Bool"(error in=w398, "DisabledEnum"=w397) -> (error out=w396:errorcluster)  [unwired: 1 in, 1 out]
              }
              event "Stop": Value Change {
                n186 = event-data() -> ()  [unwired: 1 in, 6 out]
              }
              event User Event {
                n187 = event-data() -> ()  [unwired: 1 in, 5 out]
              }
            }
            n188 = Bundle By Name(cluster=w198, "Event Ref"=w194) -> (w195:T5)
          }
          frame "HMI: List Disable" {
            (unwired) u32[] [0] ("Index Values")
            # "Enable/Disable list of All HMI Module/List HMI if list is selected."
            n189 = Unbundle By Name(w454) -> ("HMI.List From"=w441:enum16{"All HMI", "List HMI"})
            n190 = control-ref of="HMI: List"() -> (w447:refnum<vi>)
            n191 = control-ref of="HMI: All Module"() -> (w448:refnum<vi>)
            n192 = Build Array(w447, w448) -> (w452:refnum<vi>[])
            n193 = Equal To 0?(x=w441) -> (x = 0?=w438:bool)
            n194 = Reverse 1D Array(array=w452) -> (reversed array=w451:refnum<vi>[])
            n195 = Select(t=w452, s=w438, f=w451) -> (s? t:f=w453:refnum<vi>[])
            n196 = Index Array(array=w453) -> (element #1=w450:refnum<vi>, element #2=w449:refnum<vi>)  [unwired: 2 in]
            n197 = property class="Arr (strict)" props=["Value", "Index Values"](reference=w449, error in=w439) -> (error out=w444:errorcluster, "Value"=w443:cluster{"Module Name":string, "Selected":bool}[])  [unwired: 2 out]
            n198 = for {
              tunnel: w443 -> [w472] mode=indexing
              tunnel: w444 -> [w471]
              tunnel: [w471] -> w442
              tunnel: [w470] -> w431 mode=indexing
              tunnel: [w470] -> w434 mode=indexing if=w470
              n199 = Unbundle By Name(w472) -> ("Selected"=w470:bool)
            }
            n200 = Empty Array?(array=w431) -> (empty?=w429:bool)
            n201 = Or Array Elements(Boolean array=w431) -> (logical OR=w435:bool)
            n202 = And Array Elements(Boolean array=w431) -> (logical AND=w432:bool)
            n203 = Not(x=w429) -> (.not. x?=w428:bool)
            n204 = case shown="True" w435 {
              tunnel: w442 -> [w459 w468]
              tunnel: [w459 w463] -> w445
              tunnel: [T13."Enabled" ("Disabled") T13."Disabled and Grayed Out" ("Disabled")] -> w446
              tunnel: w450 -> [w457 w461]
              tunnel: [w457 w460] -> w437
              frame False {
              }
              frame True {
                n205 = property class="Arr (strict)"(reference=w461, error in=w468) -> (reference out=w462:refnum<vi>, error out=w467:errorcluster, "Value"=w464:cluster{"Module Name":string, "Selected":bool}[])
                n206 = call "List - Reset Value.vi"("Error In"=w467, "List In"=w464) -> ("Error Out"=w466:errorcluster, "List Out"=w465:cluster{"Name":string, "Selected":bool}[])  [unwired: 8 in]
                n207 = property class="Arr (strict)"(reference=w462, error in=w466, "Value"=w465) -> (reference out=w460:refnum<vi>, error out=w463:errorcluster)
              }
            }
            n208 = Bundle By Name(cluster=w454, "HMI.List Select"=w434) -> (w436:T5)
            n209 = And(x=w432, y=w428) -> (x .and. y?=w430:bool)
            n210 = local write "HMI: Select All Module"(w430) -> ()
            n211 = property class="Arr (strict)"(reference=w437, error in=w445, "DisabledEnum"=w446, "Index Values"=u32[] [0]) -> (error out=w440:errorcluster)  [unwired: 1 out]
          }
          frame "HMI: Button Disable" {
            w478 = T13."Disabled and Grayed Out" ("new element/subarray")
            w486 = T18 [enum."Disabled and Grayed Out", enum."Disabled and Grayed Out", enum."Disabled and Grayed Out", enum."Disabled and Grayed Out", enum."Disabled and Grayed Out"] items=["Enabled", "Disabled", "Disabled and Grayed Out"] ("Disabled")
            w491 = T18 [enum."Enabled", enum."Disabled and Grayed Out", enum."Disabled and Grayed Out", enum."Disabled and Grayed Out", enum."Disabled and Grayed Out"] items=["Enabled", "Disabled", "Disabled and Grayed Out"] ("Disabled")
            # "Enable/Disable button"
            n212 = Unbundle By Name(w495) -> ("HMI.Button Ref"=w493:refnum<vi>[], "HMI.List Select"=w484:bool[], "HMI.List From"=w494:enum16{"All HMI", "List HMI"})
            n213 = local read "HMI: Select List"() -> (w490:T4)
            n214 = case shown="\"2 Default Run Module\"..\"6 Page List: Level 3\"" w490 {
              tunnel: [w500 w502] -> w488
              tunnel: w489 -> [w500 w502]
              tunnel: [w499 w501] -> w476
              frame "1 All Module", Default {
                w499 = T18 [enum."Disabled and Grayed Out", enum."Enabled", enum."Enabled", enum."Enabled", enum."Enabled"] items=["Enabled", "Disabled", "Disabled and Grayed Out"] ("Disabled")
              }
              frame "2 Default Run Module".."6 Page List: Level 3" {
                w501 = T18 [enum."Disabled and Grayed Out", enum."Enabled", enum."Disabled and Grayed Out", enum."Enabled", enum."Enabled"] items=["Enabled", "Disabled", "Disabled and Grayed Out"] ("Disabled")
              }
            }
            n215 = Equal To 0?(x=w494) -> (x = 0?=w492:bool)
            n216 = Replace Array Subset(array=w476, new element #1=w478, index #1=3 ("index"), new element #2=w478, index #2=4 ("index")) -> (w477:T18)
            n217 = Array Size(array=w484) -> (size(s)=w483:i32)
            n218 = Or Array Elements(Boolean array=w484) -> (logical OR=w485:bool)
            n219 = Less Or Equal?(x=w483, y=1) -> (x <= y?=w481:bool)
            n220 = Not(x=w485) -> (.not. x?=w487:bool)
            n221 = Select(t=w476, s=w481, f=w477) -> (s? t:f=w475:T18)
            n222 = Select(t=w491, s=w492, f=w475) -> (s? t:f=w474:T18)
            n223 = Select(t=w486, s=w487, f=w474) -> (s? t:f=w473:T18)
            n224 = for {
              shift-right: [w506] -> w496
              shift-left: w488 -> [w507]
              tunnel: w493 -> [w505] mode=indexing
              tunnel: [w504] -> _ mode=indexing
              tunnel: w473 -> [w503] mode=indexing
              n225 = property class="Bool"(reference=w505, error in=w507, "DisabledEnum"=w503) -> (reference out=w504:refnum<vi>, error out=w506:errorcluster)
            }
          }
          frame "HMI: Update List" {
            # "Update list of HMI Module depending on Select List value"
            n226 = local read "HMI: Select List"() -> (w521:T4)
            n227 = In Range and Coerce(upper limit=Header_-_Select_List_Module."13 Button Text", x=w521, lower limit=Header_-_Select_List_Module."2 Default Run Module") -> (In Range?=w535:bool)  [unwired: 1 out]
            n228 = Select(t=w521, s=w535, f=Header_-_Select_List_Module."2 Default Run Module") -> (s? t:f=w513:T4)
            n229 = property on="HMI: Select List" class="Enum (strict)"(error in=w529, "Value"=w513) -> (error out=w511:errorcluster)  [unwired: 1 in, 1 out]
            n230 = case shown="\"9 Acquire Enable Page\"" w513 {
              tunnel: [Header_-_Select_List_Module."2 Default Run Module" ("f") Header_-_Select_List_Module."1 All Module" ("f") Header_-_Select_List_Module."3 Page Module" ("f") Header_-_Select_List_Module."3 Page Module" ("f")] -> w512
              tunnel: w511 -> [w541 w544 w547 w550]
              tunnel: [w541 w544 w547 w550] -> w510
              tunnel: [T13."Disabled and Grayed Out" ("Disabled") T13."Disabled and Grayed Out" ("Disabled") T13."Enabled" ("Disabled") T13."Enabled" ("Disabled")] -> w508
              frame "1 All Module", Default {
              }
              frame "2 Default Run Module" {
              }
              frame "9 Acquire Enable Page" {
              }
              frame "10 Log Enable Page" {
              }
            }
            n231 = property on="HMI: Default" class="Bool"(error in=w510, "DisabledEnum"=w508) -> (error out=w509:errorcluster)  [unwired: 1 in, 1 out]
            n232 = property on="Page List" class="MCListbox (strict)"(error in=w509) -> (error out=w516:errorcluster, "ItemNames"=w536:string[][])  [unwired: 1 in, 1 out]
            n233 = To Long Integer(number=w512) -> (32bit integer=w520:i32)
            n234 = To Long Integer(number=w513) -> (32bit integer=w519:i32)
            n235 = Index Array(array=w536, index (col) #1=w520, index (col) #2=w519) -> (element #1=w517:string[], element #2=w518:string[])  [unwired: 2 in]
            n236 = call "Gen - Remove Empty String Array.vi"("Data Array"=w517) -> ("Data Out"=w522:string[])  [unwired: 10 in]
            n237 = call "Gen - Remove Empty String Array.vi"("Data Array"=w518) -> ("Data Out"=w527:string[])  [unwired: 10 in]
            n238 = call "List - Set Value to All.vi"("Error In"=w516, "List In"=w522) -> ("Error Out"=w524:errorcluster, "List Out"=w523:cluster{"Name":string, "Selected":bool}[])  [unwired: 8 in]
            n239 = local read "HMI: Select List"() -> (w528:T4)
            n240 = property on="HMI: All Module" class="Arr (strict)"(error in=w524, "Value"=w523) -> (error out=w515:errorcluster)  [unwired: 1 in, 1 out]
            n241 = case shown="\"1 All Module\", Default" w528 {
              tunnel: [w552 w556] -> w526
              tunnel: w527 -> [w553 w556]
              tunnel: w515 -> [w554 w555]
              tunnel: [w554 w555] -> w525
              frame "1 All Module", Default {
                n242 = Sort 1D Array(array=w553) -> (sorted array=w552:string[])
              }
              frame "2 Default Run Module".."6 Page List: Level 3" {
              }
            }
            n243 = call "List - Set Value to All.vi"("Error In"=w525, "List In"=w526) -> ("Error Out"=w534:errorcluster, "List Out"=w533:cluster{"Name":string, "Selected":bool}[])  [unwired: 8 in]
            n244 = property on="HMI: List" class="Arr (strict)"(error in=w534, "Value"=w533) -> (error out=w530:errorcluster)  [unwired: 1 in, 1 out]
          }
          frame "HMI: Update Text Button" {
            w564 = ""
            # "Update text button for Page Selection at HMI"
            n245 = property on="Table: Button Text" class="MCListbox (strict)"(error in=w580) -> (error out=w585:errorcluster, "ItemNames"=w562:string[][], "SelectedCell"=w584:T10)  [unwired: 1 in, 1 out]
            n246 = Unbundle By Name(w584) -> ("Row"=w569:i32)
            n247 = Index Array(array=w562, index (col)=0 ("disabled index (col)")) -> (element=w561:string[])  [unwired: 1 in]
            n248 = Increment(x=w569) -> (x+1=w570:i32)
            n249 = call "Gen - Convert Int32 to String.vi"("Num In"=w570) -> ("String Out"=w572:string)  [unwired: 10 in]
            n250 = Concatenate Strings("Button ", w572) -> (w571:string)
            n251 = Empty String/Path?(string/path="Text") -> (empty?=w578:bool)
            n252 = Empty String/Path?(string/path="Tip Strip") -> (empty?=w576:bool)
            n253 = Select(t=w571, s=w578, f="Text") -> (s? t:f=w577:string)
            n254 = Select(t=w571, s=w576, f="Tip Strip") -> (s? t:f=w574:string)
            n255 = Equal?(x=w561, y="Text") -> (x = y?=w559:bool[])
            n256 = To Upper Case(1:w577) -> (0:w583:string)
            n257 = Or Array Elements(Boolean array=w559) -> (logical OR=w558:bool)
            n258 = Replace Array Subset(array=w562, new element #1=w583, index (row) #1=w569, index (col) #1=0 ("disabled index (col)"), new element #2=w574, index (row) #2=w569, index (col) #2=1 ("disabled index (col)")) -> (w579:string[][])
            n259 = case shown="True" w558 {
              tunnel: w585 -> [w593 w611]
              tunnel: w579 -> [w591 _]
              tunnel: [w589 w605] -> w568
              frame False {
                n260 = property on="Table: Button Text" class="MCListbox (strict)"(error in=w593, "ItemNames"=w591, "Value"=-1 ("Table: Button Text")) -> (error out=w592:errorcluster)  [unwired: 1 in, 1 out]
                n261 = property on="Page List" class="MCListbox (strict)"(error in=w592) -> (error out=w601:errorcluster, "ItemNames"=w602:string[][])  [unwired: 1 in, 1 out]
                n262 = Index Array(array=w591, index (col) #1=0 ("disabled index (col)"), index (col) #2=1 ("index (col)")) -> (element #1=w595:string[], element #2=w594:string[])  [unwired: 2 in]
                n263 = To Long Integer(number=Header_-_Select_List_Module."13 Button Text" ("Select List Module")) -> (32bit integer=w600:i32)
                n264 = To Long Integer(number=Header_-_Select_List_Module."14 Button Tip Strip" ("Select List Module")) -> (32bit integer=w597:i32)
                n265 = Replace Array Subset(array=w602, new element #1=w595, index (col) #1=w600, new element #2=w594, index (col) #2=w597) -> (w599:string[][])  [unwired: 2 in]
                n266 = property on="Page List" class="MCListbox (strict)"(error in=w601, "ItemNames"=w599) -> (error out=w589:errorcluster)  [unwired: 1 in, 1 out]
              }
              frame True {
                # "Same button name defined"
                n267 = call "Gen - Popup Single Button (Auto Close).vi"("Type"=enum16{"Error", "Info"}."Error", "Error in"=w611, "Auto Close? F"=TRUE, "Message in"="Cannot rename the button text because the button with that is already exists.", "Header"="Developer") -> ("Error out"=w610:errorcluster)  [unwired: 5 in, 1 out]
                n268 = call <vilib>:"Clear Errors.vi"("error in (no error)"=w610) -> ("error out"=w605:errorcluster)  [unwired: 5 in, 1 out]
              }
            }
            n269 = property on="Text" class="Str"(error in=w568, "Value"=w564) -> (error out=w567:errorcluster)  [unwired: 1 in, 1 out]
            n270 = property on="Tip Strip" class="Str"(error in=w567, "Value"=w564) -> (error out=w566:errorcluster)  [unwired: 1 in, 1 out]
            n271 = property on="HMI: Update Text" class="Bool"(error in=w566, "DisabledEnum"=T13."Disabled and Grayed Out" ("Disabled")) -> (error out=w565:errorcluster)  [unwired: 1 in, 1 out]
          }
          frame "HMI: Add to List" {
            # "Get selected module from All HMI Module, removing duplicate module and then insert into list."
            n272 = property on="HMI: List" class="Arr (strict)"(error in=w633) -> (error out=w632:errorcluster, "Value"=w631:cluster{"Module Name":string, "Selected":bool}[])  [unwired: 1 in, 1 out]
            n273 = call "List - Get Selected Value.vi"("Select"=enum16{"All", "True", "False"}."False", "Error In"=w632, "List In"=w631) -> ("Error Out"=w630:errorcluster, "List Out"=w629:string[])  [unwired: 7 in]
            n274 = property on="HMI: All Module" class="Arr (strict)"(error in=w630) -> (error out=w636:errorcluster, "Value"=w635:cluster{"Module Name":string, "Selected":bool}[])  [unwired: 1 in, 1 out]
            n275 = call "List - Get Selected Value.vi"("Select"=enum16{"All", "True", "False"}."True", "Error In"=w636, "List In"=w635) -> ("Error Out"=w625:errorcluster, "List Out"=w634:string[])  [unwired: 7 in]
            n276 = Build Array (concatenate)(w629, w634) -> (w628:string[])
            n277 = local read "HMI: Select List"() -> (w627:T4)
            n278 = call "Remove Duplicates From 1D Array.vim"("array"=w628) -> ("array with duplicates removed"=w626:string[])  [unwired: 10 in]
            n279 = case shown="\"1 All Module\", Default" w627 {
              tunnel: [w643 w647] -> w623
              tunnel: w626 -> [w644 w647]
              tunnel: w625 -> [w645 w646]
              tunnel: [w645 w646] -> w624
              frame "1 All Module", Default {
                n280 = Sort 1D Array(array=w644) -> (sorted array=w643:string[])
              }
              frame "2 Default Run Module".."6 Page List: Level 3" {
              }
            }
            n281 = call "List - Set Value to All.vi"("Error In"=w624, "List In"=w623) -> ("Error Out"=w637:errorcluster, "List Out"=w638:cluster{"Name":string, "Selected":bool}[])  [unwired: 8 in]
            n282 = property on="HMI: List" class="Arr (strict)"(error in=w637, "Value"=w638) -> (error out=w617:errorcluster)  [unwired: 1 in, 1 out]
            n283 = property on="HMI: All Module" class="Arr (strict)"(error in=w617) -> (error out=w613:errorcluster, "Value"=w616:cluster{"Module Name":string, "Selected":bool}[])  [unwired: 1 in, 1 out]
            n284 = Unbundle By Name(w640) -> ()  [unwired: 1 out]
            n285 = call "List - Get Selected Value.vi"("Select"=enum16{"All", "True", "False"}."All", "Error In"=w613, "List In"=w616) -> ("Error Out"=w612:errorcluster, "List Out"=w614:string[])  [unwired: 7 in]
            n286 = call "List - Set Value to All.vi"("Error In"=w612, "List In"=w614) -> ("Error Out"=w619:errorcluster, "List Out"=w620:cluster{"Name":string, "Selected":bool}[])  [unwired: 8 in]
            n287 = property on="HMI: All Module" class="Arr (strict)"(error in=w619, "Value"=w620, "Index Values"=u32[] [0]) -> (error out=w639:errorcluster)  [unwired: 1 in, 1 out]
          }
          frame "HMI: Remove from List" {
            # "Remove selected module from list"
            n288 = property on="HMI: List" class="Arr (strict)"(error in=w657) -> (error out=w661:errorcluster, "Value"=w658:cluster{"Module Name":string, "Selected":bool}[])  [unwired: 1 in, 1 out]
            n289 = local read "HMI: Select List"() -> (w656:T4)
            n290 = call "List - Get Selected Value.vi"("Select"=enum16{"All", "True", "False"}."False", "Error In"=w661, "List In"=w658) -> ("Error Out"=w655:errorcluster, "List Out"=w653:string[])  [unwired: 7 in]
            n291 = case shown="\"1 All Module\", Default" w656 {
              tunnel: [w665 w669] -> w652
              tunnel: w653 -> [w666 w669]
              tunnel: w655 -> [w667 w668]
              tunnel: [w667 w668] -> w654
              frame "1 All Module", Default {
                n292 = Sort 1D Array(array=w666) -> (sorted array=w665:string[])
              }
              frame "2 Default Run Module".."6 Page List: Level 3" {
              }
            }
            n293 = call "List - Set Value to All.vi"("Error In"=w654, "List In"=w652) -> ("Error Out"=w660:errorcluster, "List Out"=w659:cluster{"Name":string, "Selected":bool}[])  [unwired: 8 in]
            n294 = property on="HMI: List" class="Arr (strict)"(error in=w660, "Value"=w659) -> (error out=w650:errorcluster)  [unwired: 1 in, 1 out]
            n295 = property on="HMI: Select All Module" class="Bool (strict)"(error in=w650, "Value"=FALSE ("HMI: Select All Module")) -> (error out=w649:errorcluster)  [unwired: 1 in, 1 out]
          }
          frame "HMI: Sort List" {
            # "Sort the list alphabetically."
            n296 = property on="HMI: List" class="Arr (strict)"(error in=w675) -> (error out=w671:errorcluster, "Value"=w673:cluster{"Module Name":string, "Selected":bool}[])  [unwired: 1 in, 1 out]
            n297 = for {
              tunnel: w671 -> [w683]
              tunnel: w673 -> [w684] mode=indexing
              tunnel: [w683] -> w670
              tunnel: [w682] -> w672 mode=indexing
              n298 = Unbundle(w684) -> ("Module Name"=w682:string)  [unwired: 1 out]
            }
            n299 = Sort 1D Array(array=w672) -> (sorted array=w677:string[])
            n300 = call "List - Set Value to All.vi"("Error In"=w670, "List In"=w677) -> ("Error Out"=w678:errorcluster, "List Out"=w676:cluster{"Name":string, "Selected":bool}[])  [unwired: 8 in]
            n301 = property on="HMI: List" class="Arr (strict)"(error in=w678, "Value"=w676) -> (error out=w674:errorcluster)  [unwired: 1 in, 1 out]
          }
          frame "HMI: Up List" {
            # "Increase row index of selected module by 1"
            n302 = property on="HMI: List" class="Arr (strict)"(error in=w695) -> (error out=w696:errorcluster, "Value"=w697:cluster{"Module Name":string, "Selected":bool}[])  [unwired: 1 in, 1 out]
            n303 = call "List - Get First Selected Value.vi"("Error In"=w696, "List In"=w697) -> ("Error Out"=w688:errorcluster, "Index"=w694:i32, "List Out"=w693:string[])  [unwired: 7 in]
            n304 = Decrement(x=w694) -> (x-1=w689:i32)
            n305 = Index Array(array=w693, index=w694) -> (element=w692:string)
            n306 = Insert Into Array(array=w693, index=w689, new element=w692) -> (w691:string[])
            n307 = call "Remove Duplicates From 1D Array.vim"("array"=w691) -> ("array with duplicates removed"=w690:string[])  [unwired: 10 in]
            n308 = call "List - Up Index.vi"("Error In"=w688, "Index"=w689, "List In"=w690) -> ("Error Out"=w686:errorcluster, "List Out"=w687:cluster{"Name":string, "Selected":bool}[])  [unwired: 7 in]
            n309 = property on="HMI: List" class="Arr (strict)"(error in=w686, "Value"=w687) -> (error out=w685:errorcluster)  [unwired: 1 in, 1 out]
          }
          frame "HMI: Down List" {
            # "Increase row index of selected module by 1"
            n310 = property on="HMI: List" class="Arr (strict)"(error in=w714) -> (error out=w718:errorcluster, "Value"=w719:cluster{"Module Name":string, "Selected":bool}[])  [unwired: 1 in, 1 out]
            n311 = call "List - Get First Selected Value.vi"("Error In"=w718, "List In"=w719) -> ("Error Out"=w717:errorcluster, "Index"=w709:i32, "List Out"=w708:string[])  [unwired: 7 in]
            n312 = Array Size(array=w708) -> (size(s)=w702:i32)
            n313 = Decrement(x=w702) -> (x-1=w701:i32)
            n314 = Increment(x=w709) -> (x+1=w706:i32)
            n315 = Index Array(array=w708, index=w709) -> (element=w713:string)
            n316 = Delete From Array(array=w708, index=w709) -> (array with subset deleted=w712:string[])  [unwired: 1 in, 1 out]
            n317 = In Range and Coerce(upper limit=w701, x=w706, lower limit=0) -> (coerced(x)=w704:i32, In Range?=w705:bool)
            n318 = Select(t=w704, s=w705, f=w701) -> (s? t:f=w703:i32)
            n319 = Insert Into Array(array=w712, index=w703, new element=w713) -> (w711:string[])
            n320 = call "List - Up Index.vi"("Error In"=w717, "Index"=w703, "List In"=w711) -> ("Error Out"=w715:errorcluster, "List Out"=w716:cluster{"Name":string, "Selected":bool}[])  [unwired: 7 in]
            n321 = property on="HMI: List" class="Arr (strict)"(error in=w715, "Value"=w716) -> (error out=w710:errorcluster)  [unwired: 1 in, 1 out]
          }
          frame "HMI: Set Default List" {
            n322 = property on="HMI: List" class="Arr (strict)"(error in=w724) -> (error out=w736:errorcluster, "Value"=w735:cluster{"Module Name":string, "Selected":bool}[])  [unwired: 1 in, 1 out]
            n323 = call "List - Get Selected Value.vi"("Select"=enum16{"All", "True", "False"}."False", "Error In"=w736, "List In"=w735) -> ("Error Out"=w734:errorcluster, "List Out"=w733:string[])  [unwired: 7 in]
            n324 = property on="HMI: All Module" class="Arr (strict)"(error in=w734) -> (error out=w738:errorcluster, "Value"=w737:cluster{"Module Name":string, "Selected":bool}[])  [unwired: 1 in, 1 out]
            n325 = call "List - Get Selected Value.vi"("Select"=enum16{"All", "True", "False"}."All", "Error In"=w738, "List In"=w737) -> ("Error Out"=w730:errorcluster, "List Out"=w723:string[])  [unwired: 7 in]
            n326 = Build Array (concatenate)(w733, w723) -> ()  [unwired: 1 out]
            n327 = local read "HMI: Select List"() -> (w732:T4)
            n328 = call "Remove Duplicates From 1D Array.vim"("array"=w723) -> ("array with duplicates removed"=w731:string[])  [unwired: 10 in]
            n329 = case shown="\"2 Default Run Module\"..\"6 Page List: Level 3\"" w732 {
              tunnel: [w744 w748] -> w728
              tunnel: w731 -> [w745 w748]
              tunnel: w730 -> [w746 w747]
              tunnel: [w746 w747] -> w729
              frame "1 All Module", Default {
                n330 = Sort 1D Array(array=w745) -> (sorted array=w744:string[])
              }
              frame "2 Default Run Module".."6 Page List: Level 3" {
              }
            }
            n331 = call "List - Set Value to All.vi"("Error In"=w729, "List In"=w728) -> ("Error Out"=w739:errorcluster, "List Out"=w740:cluster{"Name":string, "Selected":bool}[])  [unwired: 8 in]
            n332 = property on="HMI: List" class="Arr (strict)"(error in=w739, "Value"=w740) -> (error out=w725:errorcluster)  [unwired: 1 in, 1 out]
          }
          frame "RT: Add to List" {
            # "Get selected module from All HMI Module, removing duplicate module and then insert into list."
            n333 = property on="RT: List" class="Arr (strict)"(error in=w758) -> (error out=w757:errorcluster, "Value"=w756:cluster{"Module Name":string, "Selected":bool}[])  [unwired: 1 in, 1 out]
            n334 = call "List - Get Selected Value.vi"("Select"=enum16{"All", "True", "False"}."False", "Error In"=w757, "List In"=w756) -> ("Error Out"=w755:errorcluster, "List Out"=w754:string[])  [unwired: 7 in]
            n335 = property on="RT: All Module" class="Arr (strict)"(error in=w755) -> (error out=w761:errorcluster, "Value"=w760:cluster{"Module Name":string, "Selected":bool}[])  [unwired: 1 in, 1 out]
            n336 = call "List - Get Selected Value.vi"("Select"=enum16{"All", "True", "False"}."True", "Error In"=w761, "List In"=w760) -> ("Error Out"=w752:errorcluster, "List Out"=w759:string[])  [unwired: 7 in]
            n337 = Build Array (concatenate)(w754, w759) -> (w753:string[])
            n338 = call "Remove Duplicates From 1D Array.vim"("array"=w753) -> ("array with duplicates removed"=w751:string[])  [unwired: 10 in]
            n339 = call "List - Set Value to All.vi"("Error In"=w752, "List In"=w751) -> ("Error Out"=w762:errorcluster, "List Out"=w763:cluster{"Name":string, "Selected":bool}[])  [unwired: 8 in]
            n340 = property on="RT: List" class="Arr (strict)"(error in=w762, "Value"=w763) -> (error out=w765:errorcluster)  [unwired: 1 in, 1 out]
            n341 = Unbundle By Name(w769) -> ("RT.All Module"=w768:string[])
            n342 = call "List - Set Value to All.vi"("Error In"=w765, "List In"=w768) -> ("Error Out"=w764:errorcluster, "List Out"=w767:cluster{"Name":string, "Selected":bool}[])  [unwired: 8 in]
            n343 = property on="RT: All Module" class="Arr (strict)"(error in=w764, "Value"=w767) -> (error out=w766:errorcluster)  [unwired: 1 in, 1 out]
          }
          frame "RT: Remove from List" {
            # "Remove selected module from list"
            n344 = property on="RT: List" class="Arr (strict)"(error in=w776) -> (error out=w780:errorcluster, "Value"=w777:cluster{"Module Name":string, "Selected":bool}[])  [unwired: 1 in, 1 out]
            n345 = call "List - Get Selected Value.vi"("Select"=enum16{"All", "True", "False"}."False", "Error In"=w780, "List In"=w777) -> ("Error Out"=w774:errorcluster, "List Out"=w773:string[])  [unwired: 7 in]
            n346 = call "List - Set Value to All.vi"("Error In"=w774, "List In"=w773) -> ("Error Out"=w779:errorcluster, "List Out"=w778:cluster{"Name":string, "Selected":bool}[])  [unwired: 8 in]
            n347 = property on="RT: List" class="Arr (strict)"(error in=w779, "Value"=w778) -> (error out=w775:errorcluster)  [unwired: 1 in, 1 out]
          }
          frame "RT: Up List" {
            # "Increase row index of selected module by 1"
            n348 = property on="RT: List" class="Arr (strict)"(error in=w794) -> (error out=w795:errorcluster, "Value"=w796:cluster{"Module Name":string, "Selected":bool}[])  [unwired: 1 in, 1 out]
            n349 = call "List - Get First Selected Value.vi"("Error In"=w795, "List In"=w796) -> ("Error Out"=w787:errorcluster, "Index"=w793:i32, "List Out"=w792:string[])  [unwired: 7 in]
            n350 = Decrement(x=w793) -> (x-1=w788:i32)
            n351 = Index Array(array=w792, index=w793) -> (element=w791:string)
            n352 = Insert Into Array(array=w792, index=w788, new element=w791) -> (w790:string[])
            n353 = call "Remove Duplicates From 1D Array.vim"("array"=w790) -> ("array with duplicates removed"=w789:string[])  [unwired: 10 in]
            n354 = call "List - Up Index.vi"("Error In"=w787, "Index"=w788, "List In"=w789) -> ("Error Out"=w785:errorcluster, "List Out"=w786:cluster{"Name":string, "Selected":bool}[])  [unwired: 7 in]
            n355 = property on="RT: List" class="Arr (strict)"(error in=w785, "Value"=w786) -> (error out=w784:errorcluster)  [unwired: 1 in, 1 out]
          }
          frame "RT: Down List" {
            # "Increase row index of selected module by 1"
            n356 = property on="HMI: List" class="Arr (strict)"(error in=w813) -> (error out=w817:errorcluster, "Value"=w818:cluster{"Module Name":string, "Selected":bool}[])  [unwired: 1 in, 1 out]
            n357 = call "List - Get First Selected Value.vi"("Error In"=w817, "List In"=w818) -> ("Error Out"=w816:errorcluster, "Index"=w808:i32, "List Out"=w807:string[])  [unwired: 7 in]
            n358 = Array Size(array=w807) -> (size(s)=w801:i32)
            n359 = Decrement(x=w801) -> (x-1=w800:i32)
            n360 = Increment(x=w808) -> (x+1=w805:i32)
            n361 = Index Array(array=w807, index=w808) -> (element=w812:string)
            n362 = Delete From Array(array=w807, index=w808) -> (array with subset deleted=w811:string[])  [unwired: 1 in, 1 out]
            n363 = In Range and Coerce(upper limit=w800, x=w805, lower limit=0) -> (coerced(x)=w803:i32, In Range?=w804:bool)
            n364 = Select(t=w803, s=w804, f=w800) -> (s? t:f=w802:i32)
            n365 = Insert Into Array(array=w811, index=w802, new element=w812) -> (w810:string[])
            n366 = call "List - Up Index.vi"("Error In"=w816, "Index"=w802, "List In"=w810) -> ("Error Out"=w814:errorcluster, "List Out"=w815:cluster{"Name":string, "Selected":bool}[])  [unwired: 7 in]
            n367 = property on="HMI: List" class="Arr (strict)"(error in=w814, "Value"=w815) -> (error out=w809:errorcluster)  [unwired: 1 in, 1 out]
          }
          frame "RT: List Disable" {
            # "Enable/Disable list of All HMI Module/List HMI if list is selected."
            n368 = Unbundle By Name(w847) -> ("RT.List From"=w835:enum16{"All RT", "List RT"})
            n369 = control-ref of="RT: List"() -> (w841:refnum<vi>)
            n370 = control-ref of="RT: All Module"() -> (w842:refnum<vi>)
            n371 = Build Array(w841, w842) -> (w845:refnum<vi>[])
            n372 = Equal To 0?(x=w835) -> (x = 0?=w833:bool)
            n373 = Reverse 1D Array(array=w845) -> (reversed array=w844:refnum<vi>[])
            n374 = Select(t=w845, s=w833, f=w844) -> (s? t:f=w846:refnum<vi>[])
            n375 = Index Array(array=w846) -> (element #1=w843:refnum<vi>, element #2=w824:refnum<vi>)  [unwired: 2 in]
            n376 = property class="Arr (strict)"(reference=w824, error in=w834, "Index Values"=u32[] [0]) -> (error out=w838:errorcluster, "Value"=w837:cluster{"Module Name":string, "Selected":bool}[])  [unwired: 1 out]
            n377 = for {
              tunnel: w837 -> [w866] mode=indexing
              tunnel: w838 -> [w865]
              tunnel: [w865] -> w836
              tunnel: [w864] -> w829 mode=indexing
              tunnel: [w864] -> w828 mode=indexing if=w864
              n378 = Unbundle By Name(w866) -> ("Selected"=w864:bool)
            }
            n379 = Or Array Elements(Boolean array=w829) -> (logical OR=w830:bool)
            n380 = case shown="False" w830 {
              tunnel: w836 -> [w852 w862]
              tunnel: [w852 w857] -> w839
              tunnel: [w850 T13."Disabled and Grayed Out" ("Disabled")] -> w840
              tunnel: w843 -> [w851 w855]
              tunnel: [w851 w854] -> w832
              tunnel: [w850 T13."Enabled" ("Disabled")] -> w823
              frame False {
                w850 = T13."Enabled" ("Disabled")
              }
              frame True {
                n381 = property class="Arr (strict)"(reference=w855, error in=w862) -> (reference out=w856:refnum<vi>, error out=w861:errorcluster, "Value"=w858:cluster{"Module Name":string, "Selected":bool}[])
                n382 = call "List - Reset Value.vi"("Error In"=w861, "List In"=w858) -> ("Error Out"=w860:errorcluster, "List Out"=w859:cluster{"Name":string, "Selected":bool}[])  [unwired: 8 in]
                n383 = property class="Arr (strict)"(reference=w856, error in=w860, "Value"=w859) -> (reference out=w854:refnum<vi>, error out=w857:errorcluster)
              }
            }
            n384 = Bundle By Name(cluster=w847, "RT.List Select"=w828) -> (w831:T5)
            n385 = property class="Arr (strict)"(reference=w832, error in=w839, "DisabledEnum"=w840, "Index Values"=u32[] [0]) -> (error out=w825:errorcluster)  [unwired: 1 out]
            n386 = property class="Arr (strict)"(reference=w824, error in=w825, "DisabledEnum"=w823) -> (error out=w822:errorcluster)  [unwired: 1 out]
          }
          frame "RT: Button Disable" {
            w881 = T18 [enum."Disabled and Grayed Out", enum."Enabled", enum."Enabled", enum."Enabled", enum."Enabled"] items=["Enabled", "Disabled", "Disabled and Grayed Out"] ("Disabled")
            w886 = T13."Disabled and Grayed Out" ("new element/subarray")
            w894 = T18 [enum."Disabled and Grayed Out", enum."Disabled and Grayed Out", enum."Disabled and Grayed Out", enum."Disabled and Grayed Out", enum."Disabled and Grayed Out"] items=["Enabled", "Disabled", "Disabled and Grayed Out"] ("Disabled")
            w896 = T18 [enum."Enabled", enum."Disabled and Grayed Out", enum."Disabled and Grayed Out", enum."Disabled and Grayed Out", enum."Disabled and Grayed Out"] items=["Enabled", "Disabled", "Disabled and Grayed Out"] ("Disabled")
            # "Enable/Disable button"
            n387 = Unbundle By Name(w899) -> ("RT.Button Ref"=w898:refnum<vi>[], "RT.List Select"=w892:bool[], "RT.List From"=w867:enum16{"All RT", "List RT"})
            n388 = local read "RT: Select All Module"() -> (w871:bool)
            n389 = local read "RT: Select All List"() -> (w870:bool)
            n390 = Equal?(x=w867, y=enum16{"All RT", "List RT"}."All RT" ("RT.List From")) -> (x = y?=w869:bool)
            n391 = And(x=w869, y=w871) -> (x .and. y?=w872:bool)
            n392 = And(x=w869, y=w870) -> (x .and. y?=w868:bool)
            n393 = Select(t=T13."Enabled" ("new element/subarray"), s=w872, f=T13."Disabled and Grayed Out" ("new element/subarray")) -> ()  [unwired: 1 out]
            n394 = Select(t=T13."Disabled and Grayed Out" ("new element/subarray"), s=w868, f=T13."Enabled" ("new element/subarray")) -> ()  [unwired: 1 out]
            n395 = property on="RT: Select All Module" class="Bool (strict)" props=["DisabledEnum"](error in=w878) -> (error out=w877:errorcluster)  [unwired: 1 in, 2 out]
            n396 = property on="RT: Select All List" class="Bool (strict)" props=["DisabledEnum"](error in=w877) -> (error out=w879:errorcluster)  [unwired: 1 in, 2 out]
            n397 = Equal To 0?(x=w867) -> (x = 0?=w897:bool)
            n398 = Replace Array Subset(array=w881, new element #1=w886, index #1=2 ("index"), new element #2=w886, index #2=3 ("index")) -> (w885:T18)
            n399 = Array Size(array=w892) -> (size(s)=w891:i32)
            n400 = Or Array Elements(Boolean array=w892) -> (logical OR=w893:bool)
            n401 = Less Or Equal?(x=w891, y=1) -> (x <= y?=w889:bool)
            n402 = Not(x=w893) -> (.not. x?=w895:bool)
            n403 = Select(t=w881, s=w889, f=w885) -> (s? t:f=w884:T18)
            n404 = Select(t=w896, s=w897, f=w884) -> (s? t:f=w883:T18)
            n405 = Select(t=w894, s=w895, f=w883) -> (s? t:f=w882:T18)
            n406 = for {
              shift-right: [w906] -> w900
              shift-left: w879 -> [w907]
              tunnel: w898 -> [w905] mode=indexing
              tunnel: [w904] -> _ mode=indexing
              tunnel: w882 -> [w903] mode=indexing
              n407 = property class="Bool"(reference=w905, error in=w907, "DisabledEnum"=w903) -> (reference out=w904:refnum<vi>, error out=w906:errorcluster)
            }
          }
          frame "Update Page List" {
            # "Update configuration into Page List"
            n408 = property on="RT: List" class="Arr (strict)"(error in=w908) -> (error out=w912:errorcluster, "Value"=w913:cluster{"Module Name":string, "Selected":bool}[])  [unwired: 1 in, 1 out]
            n409 = for {
              tunnel: w912 -> [w931]
              tunnel: w913 -> [w933] mode=indexing
              tunnel: [w931] -> w911
              tunnel: [w932] -> w909 mode=indexing
              n410 = Unbundle(w933) -> ("Module Name"=w932:string)  [unwired: 1 out]
            }
            n411 = property on="HMI: List" class="Arr (strict)"(error in=w911) -> (error out=w922:errorcluster, "Value"=w921:cluster{"Module Name":string, "Selected":bool}[])  [unwired: 1 in, 1 out]
            n412 = for {
              tunnel: w922 -> [w935]
              tunnel: w921 -> [w936] mode=indexing
              tunnel: [w935] -> w919
              tunnel: [w934] -> w920 mode=indexing
              n413 = Unbundle(w936) -> ("Module Name"=w934:string)  [unwired: 1 out]
            }
            n414 = local read "HMI: Select List"() -> (w926:T4)
            n415 = property on="Page List" class="MCListbox (strict)"(error in=w919) -> (error out=w927:errorcluster, "ItemNames"=w925:string[][])  [unwired: 1 in, 1 out]
            n416 = To Long Integer(number=w926) -> (32bit integer=w918:i32)
            n417 = Delete From Array(array=w925, index (col)=w918) -> (array with subset deleted=w924:string[][])  [unwired: 2 in, 1 out]
            n418 = To Long Integer(number=Header_-_Select_List_Module."8 Default RT Run Module" ("lower limit")) -> (32bit integer=w910:i32)
            n419 = Insert Into Array(array=w924, index (col)=w918, new element=w920) -> (w917:string[][])  [unwired: 1 in]
            n420 = Delete From Array(array=w917, index (col)=w910) -> (array with subset deleted=w916:string[][])  [unwired: 2 in, 1 out]
            n421 = Insert Into Array(array=w916, index (col)=w910, new element=w909) -> (w915:string[][])  [unwired: 1 in]
            n422 = property on="Page List" class="MCListbox (strict)"(error in=w927, "ItemNames"=w915) -> (error out=w923:errorcluster)  [unwired: 1 in, 1 out]
          }
          frame "Save Page List" {
            # "Save all configuration into file."
            n423 = property on="Page List" class="MCListbox (strict)"(error in=w957) -> (error out=w958:errorcluster, "ItemNames"=w1011:string[][])  [unwired: 1 in, 1 out]
            n424 = To Long Integer(number=Header_-_Select_List_Module."1 All Module" ("Select List Module")) -> (32bit integer=w1010:i32)
            n425 = To Long Integer(number=Header_-_Select_List_Module."2 Default Run Module" ("Select List Module")) -> (32bit integer=w1000:i32)
            n426 = To Long Integer(number=Header_-_Select_List_Module."3 Page Module" ("Select List Module")) -> (32bit integer=w999:i32)
            n427 = To Long Integer(number=Header_-_Select_List_Module."4 Page List: Level 1" ("Select List Module")) -> (32bit integer=w998:i32)
            n428 = To Long Integer(number=Header_-_Select_List_Module."5 Page List: Level 2" ("Select List Module")) -> (32bit integer=w997:i32)
            n429 = To Long Integer(number=Header_-_Select_List_Module."6 Page List: Level 3" ("Select List Module")) -> (32bit integer=w996:i32)
            n430 = To Long Integer(number=Header_-_Select_List_Module."7 All RT Module" ("Select List Module")) -> (32bit integer=w995:i32)
            n431 = To Long Integer(number=Header_-_Select_List_Module."8 Default RT Run Module" ("Select List Module")) -> (32bit integer=w994:i32)
            n432 = To Long Integer(number=Header_-_Select_List_Module."9 Acquire Enable Page" ("Select List Module")) -> (32bit integer=w993:i32)
            n433 = To Long Integer(number=Header_-_Select_List_Module."10 Log Enable Page" ("Select List Module")) -> (32bit integer=w992:i32)
            n434 = To Long Integer(number=Header_-_Select_List_Module."11 Run Page" ("Select List Module")) -> (32bit integer=w984:i32)
            n435 = To Long Integer(number=Header_-_Select_List_Module."12 Kill Page" ("Select List Module")) -> (32bit integer=w983:i32)
            n436 = To Long Integer(number=Header_-_Select_List_Module."13 Button Text" ("Select List Module")) -> (32bit integer=w982:i32)
            n437 = To Long Integer(number=Header_-_Select_List_Module."14 Button Tip Strip" ("Select List Module")) -> (32bit integer=w981:i32)
            n438 = Index Array(array=w1011, index (col) #1=w1010, index (col) #2=w1000, index (col) #3=w999, index (col) #4=w998, index (col) #5=w997, index (col) #6=w996, index (col) #7=w995, index (col) #8=w994, index (col) #9=w993, index (col) #10=w992, index (col) #11=w984, index (col) #12=w983, index (col) #13=w982, index (col) #14=w981) -> (element #1=w991:string[], element #2=w990:string[], element #3=w989:string[], element #4=w980:string[], element #5=w979:string[], element #6=w978:string[], element #7=w977:string[], element #8=w976:string[], element #9=w975:string[], element #10=w974:string[], element #11=w973:string[], element #12=w972:string[], element #13=w971:string[], element #14=w970:string[])  [unwired: 14 in]
            n439 = call "Gen - Remove Empty String Array.vi"("Data Array"=w991) -> ("Data Out"=w969:string[])  [unwired: 10 in]
            n440 = call "Gen - Remove Empty String Array.vi"("Data Array"=w990) -> ("Data Out"=w968:string[])  [unwired: 10 in]
            n441 = call "Gen - Remove Empty String Array.vi"("Data Array"=w989) -> ("Data Out"=w967:string[])  [unwired: 10 in]
            n442 = call "Gen - Remove Empty String Array.vi"("Data Array"=w980) -> ("Data Out"=w966:string[])  [unwired: 10 in]
            n443 = call "Gen - Remove Empty String Array.vi"("Data Array"=w979) -> ("Data Out"=w965:string[])  [unwired: 10 in]
            n444 = call "Gen - Remove Empty String Array.vi"("Data Array"=w978) -> ("Data Out"=w964:string[])  [unwired: 10 in]
            n445 = call "Gen - Remove Empty String Array.vi"("Data Array"=w977) -> ("Data Out"=w963:string[])  [unwired: 10 in]
            n446 = call "Gen - Remove Empty String Array.vi"("Data Array"=w976) -> ("Data Out"=w962:string[])  [unwired: 10 in]
            n447 = call "Gen - Remove Empty String Array.vi"("Data Array"=w975) -> ("Data Out"=w961:string[])  [unwired: 10 in]
            n448 = call "Gen - Remove Empty String Array.vi"("Data Array"=w974) -> ("Data Out"=w960:string[])  [unwired: 10 in]
            n449 = call "Gen - Remove Empty String Array.vi"("Data Array"=w973) -> ("Data Out"=w950:string[])  [unwired: 10 in]
            n450 = call "Gen - Remove Empty String Array.vi"("Data Array"=w972) -> ("Data Out"=w952:string[])  [unwired: 10 in]
            n451 = call "Gen - Remove Empty String Array.vi"("Data Array"=w971) -> ("Data Out"=w951:string[])  [unwired: 10 in]
            n452 = call "Gen - Remove Empty String Array.vi"("Data Array"=w970) -> ("Data Out"=w959:string[])  [unwired: 10 in]
            n453 = Bundle By Name(cluster=T14 {"HMI Configuration"={"EXE Name"="", "Project Name"="", "Max Page No"=2, "HMI State"=enum."Invalid", "Version"=enum."Demo", "Check License"=FALSE, "Font Size"=44, "Res: Height"=655, "Res: Width"=1356, "License Level"=enum."Level 2", "License Type"=enum."Perpetual"}, "All HMI Module"=["Module - DAQmx AI Daemon.vit", "Module - DAQmx AI.vi", "Module - DAQmx AO.vi", "Module - DAQmx DI.vi", "Module - DAQmx DO.vi", "Module - Error Management.vi", "Module - Login.vi", "Module - P1 Display.vi", "Module - P2 List Device.vi", "Module - P3 Configure Tags IO.vi", "Module - P4 Log Config.vi", "Module - P5 Filter.vi", "Module - P6 Calibration.vi", "Module - P7 Analysis.vi", "Module - P8 User Management.vi"], "Default HMI Module"=["Module - Error Management.vi", "Module - Login.vi", "Module - P1 Display.vi", "Module - P2 List Device.vi", "Module - P3 Configure Tags IO.vi", "Module - P4 Log Config.vi", "Module - P5 Filter.vi", "Module - P6 Calibration.vi", "Module - P7 Analysis.vi", "Module - P8 User Management.vi"], "Page Module"=["Module - P1 Display.vi", "Module - P2 List Device.vi", "Module - P3 Configure Tags IO.vi", "Module - P4 Log Config.vi", "Module - P5 Filter.vi", "Module - P6 Calibration.vi", "Module - P7 Analysis.vi", "Module - P8 User Management.vi"], "Page List: Level 1"=[], "Page List: Level 2"=[], "Page List: Level 3"=[], "All RT Module"=[], "Default RT Module"=[], "Acquire Enable Page"=[], "Log Enable Page"=[], "Run Page"=[], "Kill Page"=[], "Button"={"Text"=["MAIN", "DEVICE", "I/O SETTING", "LOGGING", "FILTER", "SCALE", "ANALYSIS", "USER", "RSVE", "RSVE"], "Tip Strip"=[]}} ("Data In"), "All HMI Module"=w969, "Default HMI Module"=w968, "Page Module"=w967, "Page List: Level 1"=w966, "Page List: Level 2"=w965, "Page List: Level 3"=w964, "All RT Module"=w963, "Default RT Module"=w962, "Acquire Enable Page"=w961, "Log Enable Page"=w960, "Run Page"=w950, "Kill Page"=w952, "Button.Text"=w951, "Button.Tip Strip"=w959) -> (w949:T14)
            n454 = local read "HMI: Check License"() -> (w944:bool)
            n455 = local read "HMI: Project Name"() -> (w940:string)
            n456 = local read "HMI: EXE Name"() -> (w939:string)
            n457 = local read "License Level"() -> (w938:T2)
            n458 = local read "HMI: Version"() -> (w943:enum16{"Demo", "User"})
            n459 = local read "License Type"() -> (w937:T3)
            n460 = local read "Res: Height"() -> (w946:i16)
            n461 = local read "Res: Width"() -> (w945:i16)
            n462 = local read "HMI State"() -> (w942:T1)
            n463 = local read "Font Size"() -> (w947:u32)
            n464 = local read "Max"() -> (w941:i32)
            n465 = Bundle By Name(cluster=w949, "HMI Configuration.EXE Name"=w939, "HMI Configuration.Project Name"=w940, "HMI Configuration.Max Page No"=w941, "HMI Configuration.HMI State"=w942, "HMI Configuration.Version"=w943, "HMI Configuration.Check License"=w944, "HMI Configuration.Font Size"=w947, "HMI Configuration.Res: Height"=w946, "HMI Configuration.Res: Width"=w945, "HMI Configuration.License Level"=w938, "HMI Configuration.License Type"=w937) -> (w948:T14)
            n466 = call "aFGV - Datalog Page.vi"("Action"=enum16{"Read", "Write"}."Write", "Error In"=w958, "Data In"=w948) -> ("Error Out"=w1015:errorcluster)  [unwired: 7 in, 1 out]
            n467 = Unbundle By Name(w1017) -> ("HMI?"=w956:bool)
            n468 = Select(t=State_-_Module_Developer."HMI: List Disable", s=w956, f=State_-_Module_Developer."RT: List Disable") -> (s? t:f=w953:T6)
          }
          frame "Load Error" {
            n469 = call "Gen - Get Application Kind.vi"("Error In"=w1020) -> ("Error Out"=w1025:errorcluster, "Application:Kind"=w1026:T15)  [unwired: 9 in]
            n470 = case shown="\"Development System\"" w1026 {
              tunnel: [w1047 w1051] -> w1023
              tunnel: [w1048 w1050] -> w1024
              tunnel: w1025 -> [w1048 w1050]
              frame "Run Time System", Default {
                w1049 = T19 2 items=["User Home"=0, "User Desktop"=1, "User Documents"=2, "User Application Data"=3, "User Preferences"=4, "User Temporary"=5, "Public Documents"=6, "Public Application Data"=7, "Public Preferences"=8, "Public Cache"=13, "System Core Libraries"=9, "System Installed Libraries"=10, "Application Files"=11, "Boot Volume Root"=12] ("system directory type")
                n471 = call <vilib>:"Get System Directory.vi"("system directory type"=w1049) -> ("system directory"=w1047:path)  [unwired: 10 in]
              }
              frame "Development System" {
                n472 = call <vilib>:"Application Directory.vi"() -> ("Application Directory"=w1053:path)
                n473 = Build Path(base path=w1053, name or relative path="HMI\\Data\\Error") -> (appended path=w1051:path)
              }
            }
            n474 = feedback #1(w1023) -> (w1029:path)
            n475 = call "File Dialog"("start path"=w1029, "prompt"="Select error file", "error in"=w1024, "pattern (all files)"="*.csv", "pattern label"="Comma Separated File") -> ("selected path"=w1021:path, "cancelled"=w1018:bool, "error out"=w1022:errorcluster)  [unwired: 7 in, 1 out]
            n476 = feedback-in #1(w1021) -> ()
            n477 = case shown="True" w1018 {
              tunnel: w1022 -> [w1044 w1046]
              tunnel: w1021 -> [w1043 _]
              tunnel: [w1034 w1045] -> w1019
              frame False {
                # "File loaded"
                n478 = call-poly <vilib>:"Read Delimited Spreadsheet.vi"("file path (dialog if empty)"=w1043, "error in (no error)"=w1044, "delimiter (\\t)"="," ("delimiter (\\t)")) -> ("all rows"=w1038:string[][], "error out"=w1040:errorcluster)  [unwired: 7 in, 4 out]
                n479 = control-ref of="Error Table"() -> (w1035:refnum<vi>)
                n480 = Delete From Array(array=w1038, index (row)=0) -> (array with subset deleted=w1037:string[][])  [unwired: 2 in, 1 out]
                n481 = call "Gen - Text Wrapper.vi"("Error In"=w1040, "Ref Listbox"=w1035, "Data in"=w1037) -> ("Error Out"=w1039:errorcluster, "Data Out"=w1041:string[][])  [unwired: 7 in]
                n482 = property on="Property Node" class="MCListbox (strict)"(reference=w1035, error in=w1039, "ItemNames"=w1041) -> (error out=w1034:errorcluster)  [unwired: 1 out]
              }
              frame True {
                n483 = call <vilib>:"Clear Errors.vi"("error in (no error)"=w1046) -> ("error out"=w1045:errorcluster)  [unwired: 5 in, 1 out]
              }
            }
          }
          frame "Close" {
            n484 = Unbundle By Name(w1055) -> ("Event Ref"=w1054:refnum<event-registration>)
            n485 = property on="Pane 2" class="Pane"(error in=w1061, "Origin"=T7 {"Horizontal"=0, "Vertical"=0}) -> (error out=w1060:errorcluster)  [unwired: 1 in, 1 out]
            n486 = Unregister For Events(event registration refnum=w1054, error in=w1060) -> (error out=w1057:errorcluster)
            n487 = property on="Tab Control" class="TabCtl (strict)"(error in=w1057, "PageSelVis"=TRUE ("Page Selector Visible"), "Position"=T8 {"Left"=16, "Top"=0}) -> (error out=w1056:errorcluster)  [unwired: 1 in, 1 out]
          }
        }
      }
      frame Error {
        n488 = call <vilib>:"Clear Errors.vi"("error in (no error)"=w1068) -> ("error out"=w1066:errorcluster)  [unwired: 5 in, 1 out]
        n489 = call "Gen - Get Application Kind.vi"("Error In"=w1066) -> ("Application:Kind"=w1065:T15)  [unwired: 9 in, 1 out]
        n490 = case shown="\"Development System\"" w1065 {
          tunnel: [w1072 w1073 w1077] -> w1067
          tunnel: w1068 -> [w1072 w1073 w1075]
          frame "invalid app kind", Default {
          }
          frame "Run Time System" {
          }
          frame "Development System" {
            n491 = call <vilib>:"Simple Error Handler.vi"("error in (no error)"=w1075) -> ("error?"=w1074:bool, "error out"=w1076:errorcluster)  [unwired: 4 in, 3 out]
            n492 = case shown="True" w1074 {
              tunnel: [w1078 w1080] -> w1077
              tunnel: w1076 -> [w1078 w1079]
              frame False {
              }
              frame True {
                n493 = call <vilib>:"Clear Errors.vi"("error in (no error)"=w1079) -> ("error out"=w1080:errorcluster)  [unwired: 5 in, 1 out]
              }
            }
          }
        }
      }
    }
    n494 = Wait (ms)(milliseconds to wait=u32 100) -> ()  [unwired: 1 out]
  }
  "Error Out" <- w3
  n495 = disable-structure shown="Disabled" {
    frame Disabled {
      n496 = call "List - Set Value to All.vi"() -> ("Error Out"=w1082:errorcluster, "List Out"=w1081:cluster{"Name":string, "Selected":bool}[])  [unwired: 10 in]
      n497 = property on="HMI: List" class="Arr (strict)"(error in=w1082, "Value"=w1081) -> ()  [unwired: 1 in, 2 out]
    }
    frame Enabled {
    }
  }
